vi "CRYGraph Polar Window.vi"() -> ()   [LabVIEW 2013]
uses:
  Control/CRYPolar Property.ctl
  Control/CRYFlag Cluster.ctl
  <vilib>/Utility/miscctls.llb/LVCursorListTypeDef.ctl
  <vilib>/Utility/miscctls.llb/LVRectTypeDef.ctl
  <vilib>/Utility/miscctls.llb/LVRowAndColumnTypeDef.ctl
  SubVI/CRYData View Global.vi
  CRYCurveLibrary/Global/CRYCurve Library Global.vi
  SubVI/CRYMain Sub Window Global.vi
panel:
  out "PhaseShow":bool=TRUE
  out "FrequencyVScrollShow":bool=TRUE
  out "LegendVScrollShow":bool=TRUE
  out "SelectedRow":i32[](array[numeric])
  out "Legend Ref":refnum<vi>
  in  "LoadFinish":bool
  in  "Legend 2":i32(listbox) caption="Legend"
  in  "AxisChange":bool
  out "MagnitudeShow":bool=TRUE
  in  "RemoveSome":bool
  in  "PaletteShow":bool
  in  "ScaleFitY 2":bool
  in  "ScaleFitY":bool
  in  "ScaleFitX":bool
  out "XY Graph Ref":refnum<vi>
  out "TotalPlotPolar":u32
  out "OldRowPolar":i32
  out "Repaint Watermark":i32
  out "PropertyTab":string
  out "Polar Plot":picture
  in  "stop":bool
  out "XYCursor":string
  in  "ColorBoxPolar":u32(colorbox)
  out "Event Name":string
  in  "Cursor":string[][](table)
  out "Queue Name":string
  out "Graph Ref":refnum<vi>
  out "Title Name":string
  out "OldRow":i32
  out "TotalPlot":u32
  out "Graph Number":i32
  in  "Frequency":i32(listbox) caption="Legend"
  out "XY Graph":cluster{"XY Graph":cluster{dbl, dbl}[]}[](graph)
  in  "OpenProperty":bool
  in  "RemoveAll":bool
  out "Test":string
  in  "ColorBox":u32(colorbox)
  in  "PropertyLoading":bool
  in  "Legend":i32[](listbox)
  in  "CursorShow":bool
  in  "LegendShow":bool
  out "Cursor Ref":refnum<vi>
  in  "StateOut":bool
  in  "XYShow":bool
  out "Polar Property":T1={"polar attributes"={"maximum"=2.0, "minimum"=0.0, "clip to min"=FALSE, "log"=FALSE, "grid color"=3381657, "plot color"=16711680, "fmt and prec"={"format"=enum."Decimal", "precision"=2}, "visible section"=4}, "Auto/Manual"=0, "Zero Adjust (deg)"=0, "Angle Increment (deg)"=0, "Mirror"=FALSE, "Auto Increment"=FALSE, "Total Rotatin (deg)"=0, "Discrete/Rannge"=0, "Show Name"=FALSE, "CurValues"=[], "CurIndex"=0, "CurColors"=[], "CurColors_Range"=[], "CurValues_Range"=[], "Pen"={"Width"=1, "Style"=enum."Solid"}, "BackgroundColor"=0} {"polar attributes"."minimum" format="%0.2f"; "polar attributes"."maximum" format="%0.2f"}
  in  "FrequencyShow":bool
  out "Frequency Ref":refnum<vi>
  in  "GraphType":string
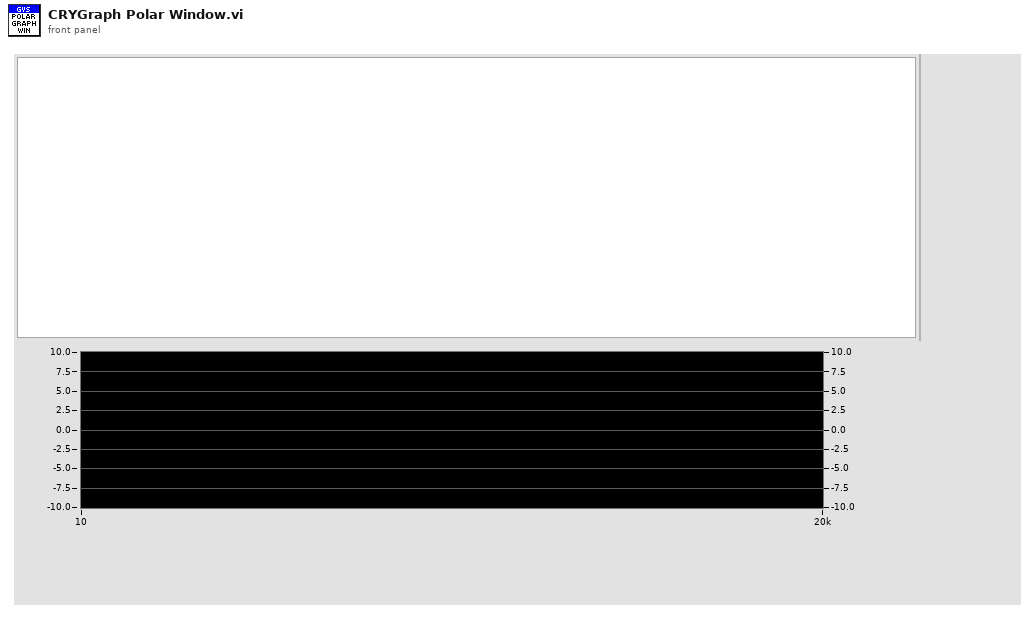
[diagram p1: front panel]
types:
  T1 = typedef "CRYPolar Property.ctl" = cluster{"polar attributes":cluster{"maximum":dbl, "minimum":dbl, "clip to min":bool, "log":bool, "grid color":u32, "plot color":u32, "fmt and prec":cluster{"format":enum8{"Decimal", "Scientific", "Engineering", "Binary", "Octal", "Hex"}, "precision":u8}, "visible section":u16}, "Auto/Manual":u16, "Zero Adjust (deg)":i32, "Angle Increment (deg)":i32, "Mirror":bool, "Auto Increment":bool, "Total Rotatin (deg)":i32, "Discrete/Rannge":u16, "Show Name":bool, "CurValues":dbl[], "CurIndex":u16, "CurColors":u32[], "CurColors_Range":u32[], "CurValues_Range":dbl[], "Pen":cluster{"Width":u16, "Style":enum32{"Solid", "Dash", "Dot", "DashDot", "DashDotDot"}}, "BackgroundColor":u32}
  T2 = typedef "CRYFlag Cluster.ctl" = cluster{"LegendShow":bool, "CellClick":bool, "Total Number":bool, "ScaleFitX":bool, "ScaleFitY":bool, "MapModeX":u8, "MapModeY":u8, "CursorShow":bool, "MagnitudeShow":bool, "PreviewShow":bool, "CursorEnabled":bool, "IntensityShow":bool, "PaletteShow":bool, "PhaseShow":bool, "XYShow":bool, "FrequencyShow":bool, "LegendVScrollShow":bool, "FrequencyVScrollShow":bool}
  T3 = enum32{"Solid", "Dash", "Dot", "DashDot", "DashDotDot"}
  T4 = enum8{"Decimal", "Scientific", "Engineering", "Binary", "Octal", "Hex"}
  T5 = typedef "LVCursorListTypeDef.ctl" = cluster{"Name":string, "Color":u32, "Style":u8, "Point Style":u8, "Name Visible":bool, "Allow Drag":bool, "Cursor Mode":u32, "Plot":i32, "Index":i32, "Position":cluster{"X":dbl, "Y":dbl}, "X Scale":u32, "Y Scale":u32, "Watch Plots":i32[], "Watch All Plots":bool, "Plot Area":i32, "Label Offset":cluster{"X":dbl, "Y":dbl}}[]
  T6 = typedef "CRYGraph Event.ctl" = cluster{"EvenName":string, "TitleName":string, "GraphName":string, "GraphType":string, "Data":variant, "Queue Name":string, "DataView Number":i32}
  T7 = typedef "LVBoundsTypeDef.ctl" = cluster{"Width":u32, "Height":u32}
  T8 = cluster{"maximum":dbl, "minimum":dbl, "clip to min":bool, "log":bool, "grid color":u32, "plot color":u32, "fmt and prec":cluster{"format":enum8{"Decimal", "Scientific", "Engineering", "Binary", "Octal", "Hex"}, "precision":u8}, "visible section":u16}
  T9 = enum16{"No Scaling", "Scale All Objects", "Scale Single Object"}
  T10 = cluster{"left":i16, "top":i16, "right":i16, "bottom":i16}
  T11 = typedef "LVRowAndColumnTypeDef.ctl" = cluster{"Row":i32, "Column":i32}
  T12 = cluster{"Name":string, "Color":u32, "Style":u8, "Point Style":u8, "Name Visible":bool, "Allow Drag":bool, "Cursor Mode":u32, "Plot":i32, "Index":i32, "Position":cluster{"X":dbl, "Y":dbl}, "X Scale":u32, "Y Scale":u32, "Watch Plots":i32[], "Watch All Plots":bool, "Plot Area":i32, "Label Offset":cluster{"X":dbl, "Y":dbl}}
  T13 = typedef "LVRectTypeDef.ctl" = cluster{"Left":i16, "Top":i16, "Right":i16, "Bottom":i16}
  T14 = typedef "LVPoint32TypeDef.ctl" = cluster{"Horizontal":i32, "Vertical":i32}
  T15 = typedef "LVPositionTypeDef.ctl" = cluster{"Left":i32, "Top":i32}
  T16 = typedef "CRYData Cluster.ctl" = cluster{"Name":string, "Curve":cluster{"x":dbl, "y":dbl, "z":dbl}[], "X data":u16, "Y data":u16, "Z data":u16, "X axis":u16, "Y axis":u16, "Z axis":u16, "X unit":string, "Y unit":string, "Z unit":string, "X dB ref":dbl, "Y dB ref":dbl, "Z dB ref":dbl, "single val":bool, "protected":bool, "display X":bool, "display Y":bool, "display Z":bool, "Test Info":string, "Step No.":i32, "Plot Settings":cluster{"Color":u32, "Interpolation":u8, "Point Style":u8, "Line Style":u8, "Point Color":u32, "Line Width":u8, "Bar Plot Style":u8, "Fill To":i16}, "AutoProtect":bool}
  T17 = cluster{"Name":string, "Color":u32, "Style":u8, "Point Style":u8, "Name Visible":bool, "Allow Drag":bool, "Cursor Mode":u32, "Plot":i32, "Index":i32, "Position":cluster{"X":dbl, "Y":dbl}, "X Scale":u32, "Y Scale":u32, "Watch Plots":i32[], "Watch All Plots":bool, "Plot Area":i32, "Label Offset":cluster{"X":dbl, "Y":dbl}}[]
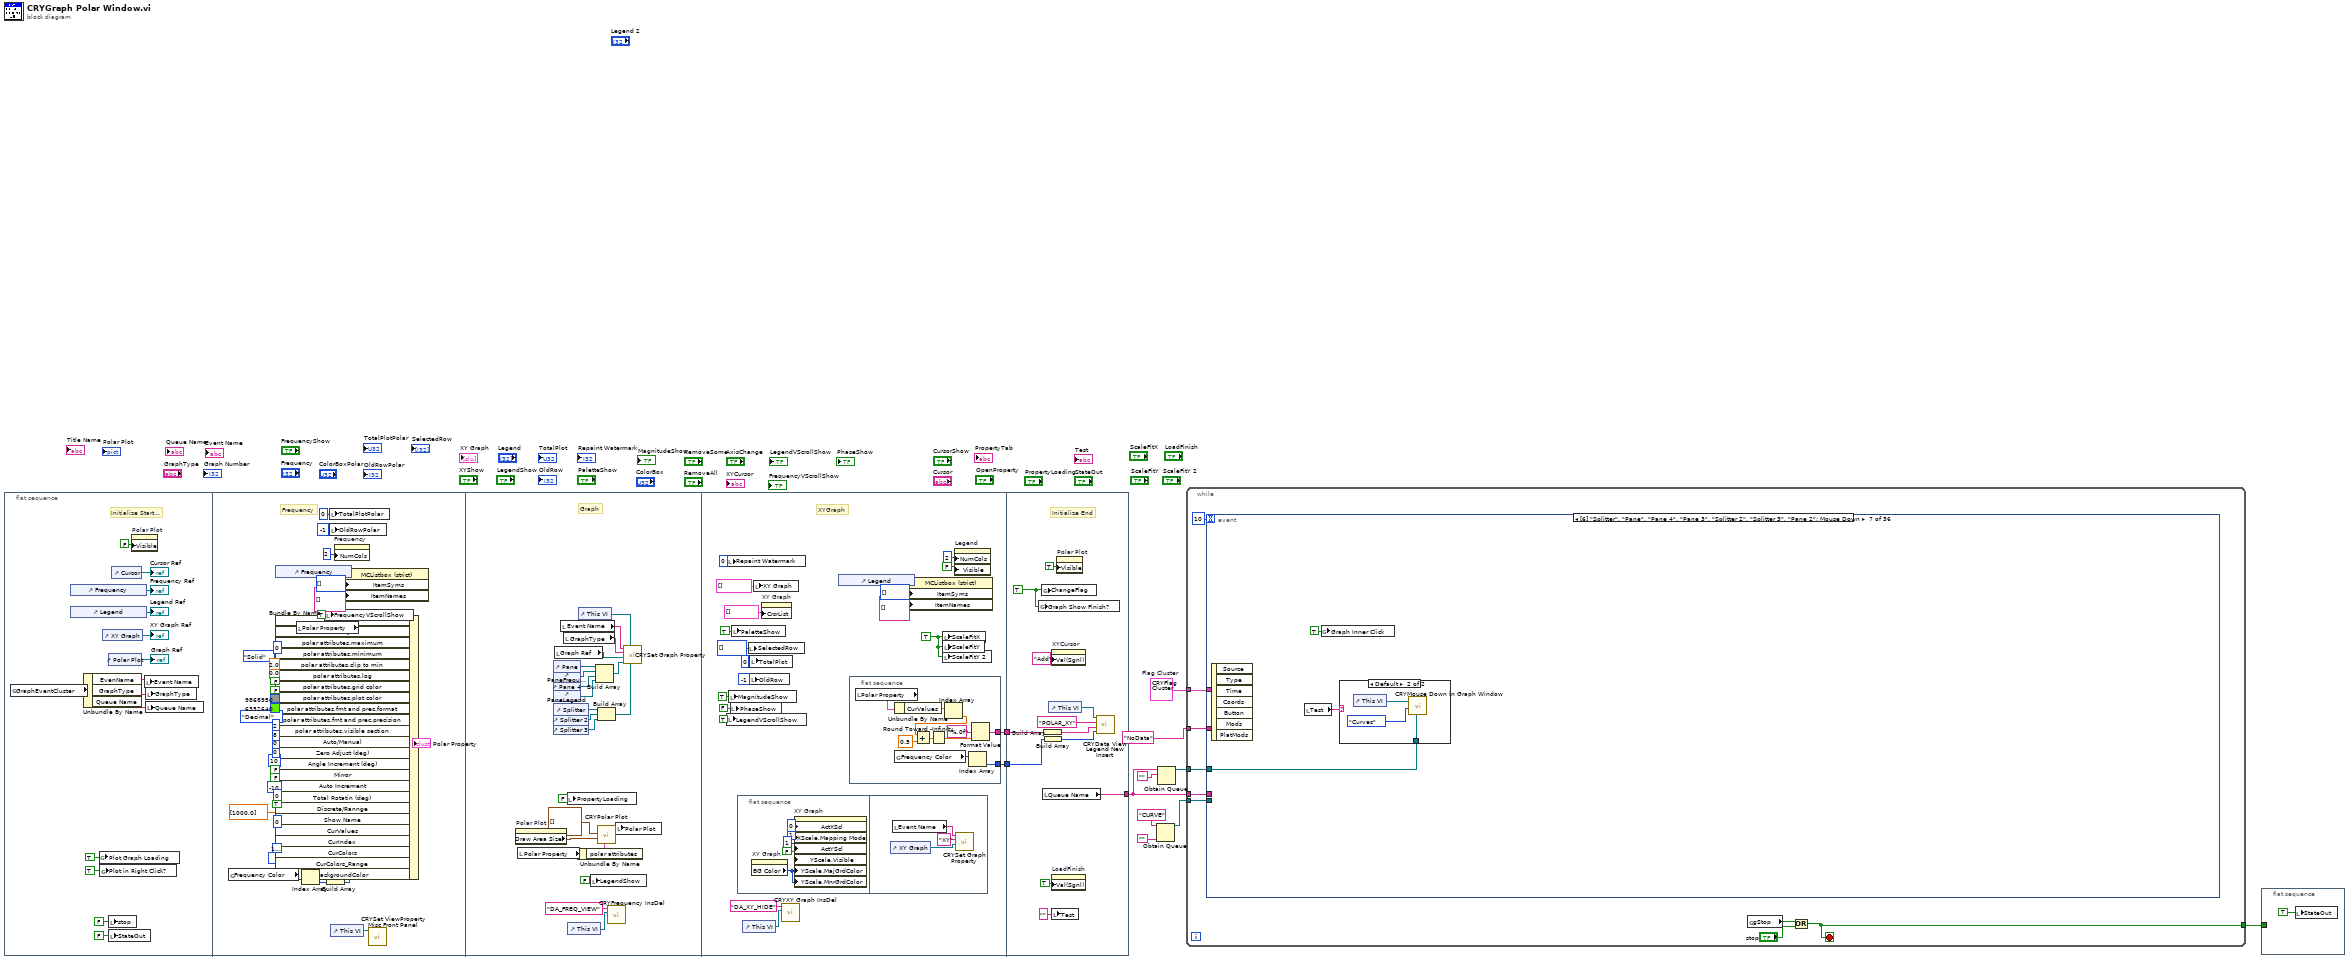
[diagram p0: block diagram]
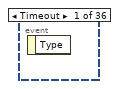
[diagram p2: hidden frame]
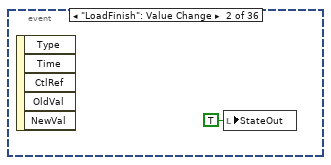
[diagram p3: hidden frame]
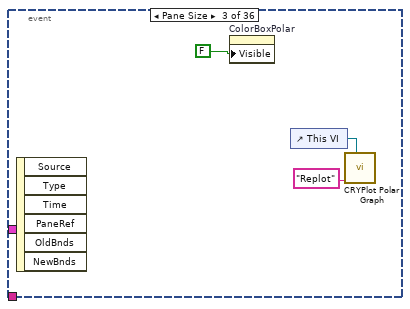
[diagram p4: hidden frame]
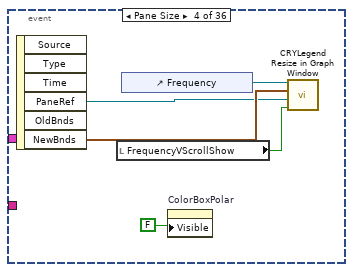
[diagram p5: hidden frame]
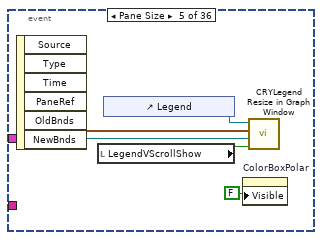
[diagram p6: hidden frame]
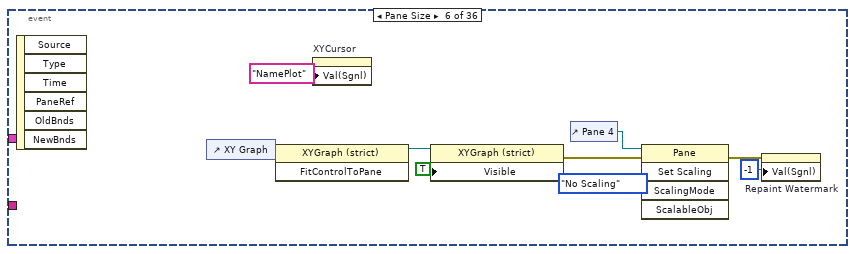
[diagram p7: hidden frame]
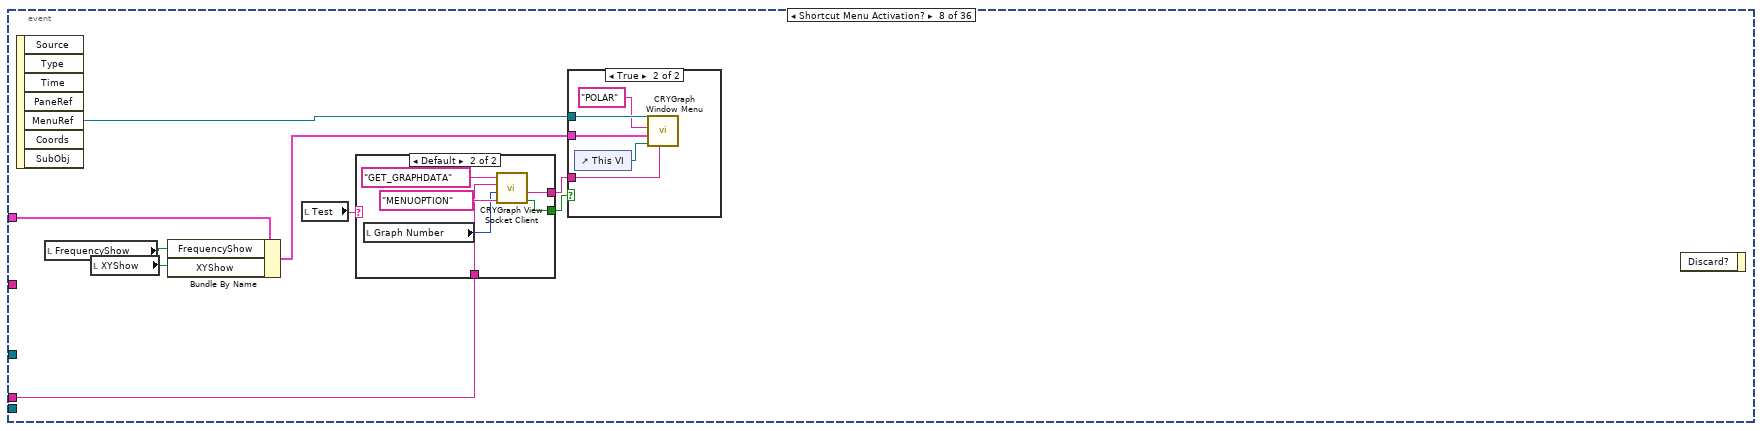
[diagram p9: hidden frame]
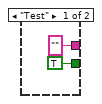
[diagram p10: hidden frame]
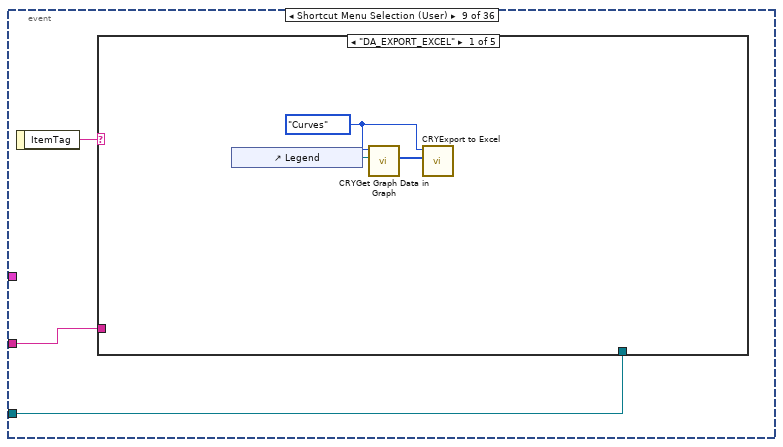
[diagram p12: hidden frame]
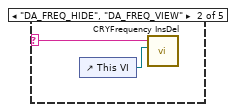
[diagram p13: hidden frame]
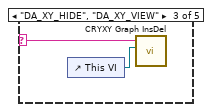
[diagram p14: hidden frame]
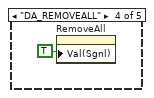
[diagram p15: hidden frame]
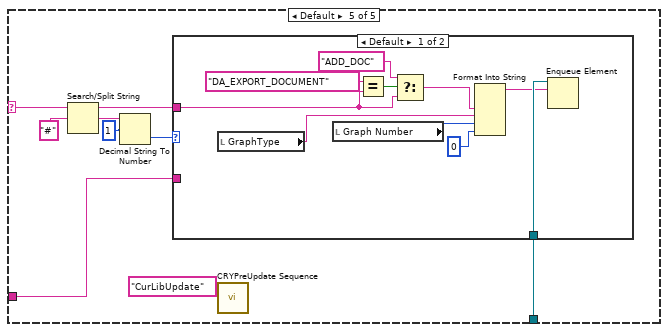
[diagram p16: hidden frame]
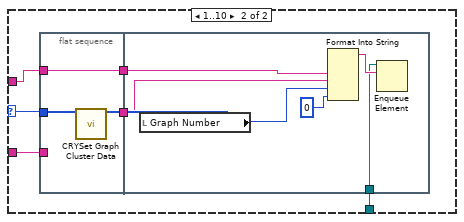
[diagram p17: hidden frame]
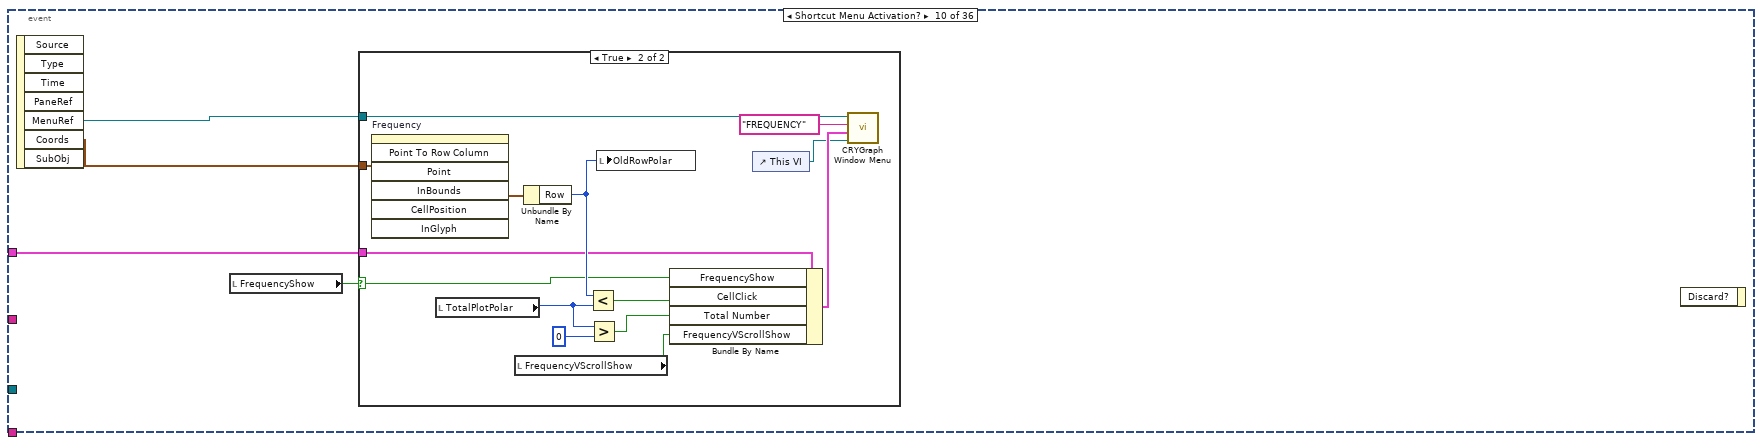
[diagram p18: hidden frame]
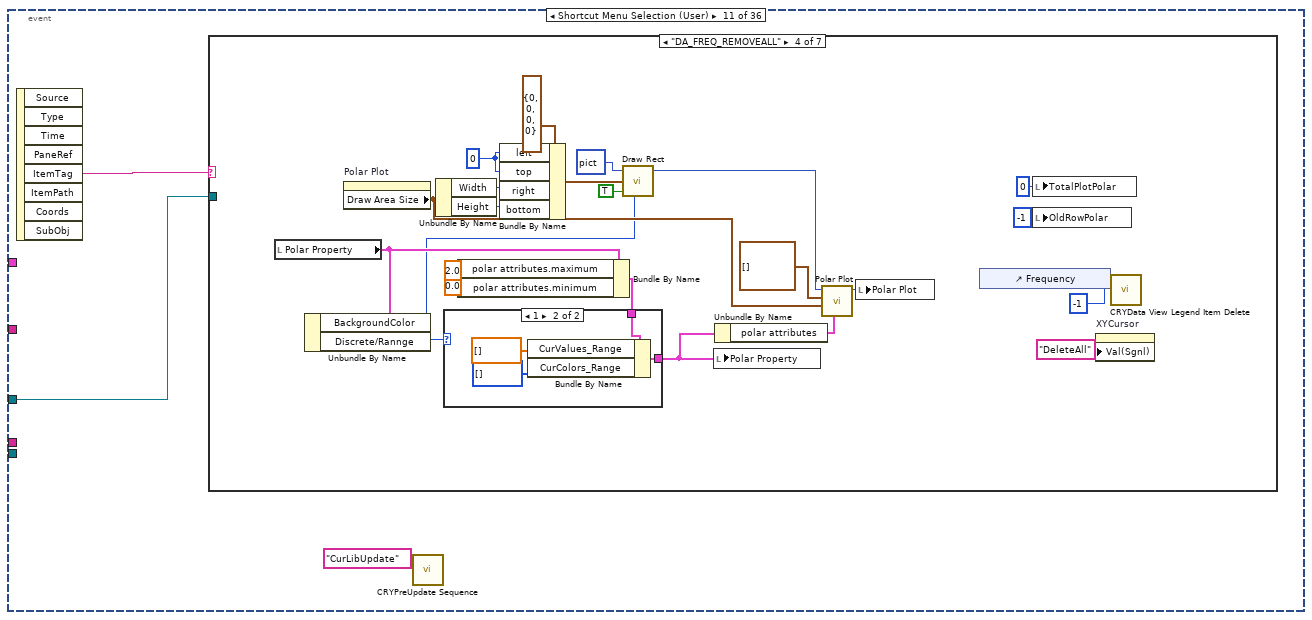
[diagram p20: hidden frame]
diagram:
  w9 = T2 {"LegendShow"=FALSE, "CellClick"=FALSE, "Total Number"=FALSE, "ScaleFitX"=FALSE, "ScaleFitY"=FALSE, "MapModeX"=0, "MapModeY"=0, "CursorShow"=FALSE, "MagnitudeShow"=FALSE, "PreviewShow"=FALSE, "CursorEnabled"=FALSE, "IntensityShow"=FALSE, "PaletteShow"=FALSE, "PhaseShow"=FALSE, "XYShow"=FALSE, "FrequencyShow"=FALSE, "LegendVScrollShow"=FALSE, "FrequencyVScrollShow"=FALSE}  # Flag Cluster
  n1 = flat-sequence {
    tunnel: [w87] -> w5
    tunnel: [w86] -> w4
    tunnel: [w129] -> w6
    tunnel: w5 -> [w127]
    tunnel: w4 -> [w125]
    frame #0 {
      # "Initialize Start..."
      n2 = global read "CRYData View Global.vi" "GraphEventCluster"() -> (w17:T6)
      n3 = control-ref of="Frequency"() -> (→"Frequency Ref":refnum<vi>)
      n4 = control-ref of="Legend"() -> (→"Legend Ref":refnum<vi>)
      n5 = Unbundle By Name(w17) -> ("EvenName"=w13:string, "GraphType"=w16:string, "Queue Name"=w18:string)
      n6 = global write "CRYData View Global.vi" "Plot Graph Loading"(TRUE ("Sequence Change for Replot")) -> ()
      n7 = global write "CRYData View Global.vi" "Plot in Right Click?"(TRUE ("Plot in Right Click?")) -> ()
      n8 = control-ref of="XY Graph"() -> (→"XY Graph Ref":refnum<vi>)
      n9 = control-ref of="Polar Plot"() -> (→"Graph Ref":refnum<vi>)
      n10 = local write "stop"(FALSE ("stop")) -> ()
      n11 = local write "StateOut"(FALSE ("StateOut")) -> ()
      n12 = control-ref of="Cursor"() -> (→"Cursor Ref":refnum<vi>)
      n13 = property on="Polar Plot" class="Pict"("Visible"=FALSE) -> ()  [unwired: 2 in, 2 out]
      n14 = local write "Event Name"(w13) -> ()
      n15 = local write "GraphType"(w16) -> ()
      n16 = local write "Queue Name"(w18) -> ()
    }
    frame #1 {
      # "Frequency"
      n17 = global read "CRYCurve Library Global.vi" "Frequency Color"() -> (w49:u32[])
      n18 = control-ref of="Frequency"() -> (w57:refnum<vi>)
      n19 = local read "Polar Property"() -> (w29:T1)
      n20 = Index Array(array=w49) -> (element=w50:u32)  [unwired: 1 in]
      n21 = local write "FrequencyVScrollShow"(TRUE ("FrequencyVScrollShow")) -> ()
      n22 = Build Array(w50) -> (w51:u32[])
      n23 = Bundle By Name(cluster=w29, "Pen.Width"=u16 0, "Pen.Style"=T3."Solid", "polar attributes.maximum"=2.0, "polar attributes.minimum"=0.0, "polar attributes.clip to min"=FALSE, "polar attributes.log"=FALSE, "polar attributes.grid color"=u32 9868950 ("grid color"), "polar attributes.plot color"=u32 6352640 ("plot color"), "polar attributes.fmt and prec.format"=T4."Decimal", "polar attributes.fmt and prec.precision"=u8 2, "polar attributes.visible section"=u16 8, "Auto/Manual"=u16 0, "Zero Adjust (deg)"=0, "Angle Increment (deg)"=10, "Mirror"=FALSE, "Auto Increment"=FALSE, "Total Rotatin (deg)"=-10, "Discrete/Rannge"=u16 0, "Show Name"=TRUE, "CurValues"=dbl[] [1000.0], "CurIndex"=u16 0, "CurColors"=w51, "CurColors_Range"=w51, "BackgroundColor"=u32 16777222 ("grid color")) -> (→"Polar Property":T1)
      n24 = local write "TotalPlotPolar"(u32 0 ("TotalPlotXY")) -> ()
      n25 = local write "OldRowPolar"(-1 ("OldRowXY")) -> ()
      n26 = control-ref of="This VI"() -> (w56:refnum<vi>)
      n27 = property on="Frequency" class="MCListbox (strict)"("NumCols"=u32 2 ("Number of Columns")) -> ()  [unwired: 2 in, 2 out]
      n28 = property on="Property Node" class="MCListbox (strict)"(reference=w57, "ItemSyms"=i32[] [] ("Item Symbols"), "ItemNames"=string[][] [] ("Item Names")) -> ()  [unwired: 1 in, 2 out]
      n29 = call "CRYSet ViewProperty Misc Front Panel.vi"("Vi Ref"=w56) -> ()  [unwired: 11 in]
    }
    frame #2 {
      # "Graph"
      n30 = property on="Polar Plot" class="Pict"() -> ("Draw Area Size"=w78:T7)  [unwired: 2 in, 2 out]
      n31 = local read "Polar Property"() -> (w82:T1)
      n32 = control-ref of="Pane"() -> (w67:refnum<vi>)
      n33 = control-ref of="PaneFrequency"() -> (w68:refnum<vi>)
      n34 = control-ref of="Pane 4"() -> (w71:refnum<vi>)
      n35 = control-ref of="PaneLegend"() -> (w72:refnum<vi>)
      n36 = control-ref of="Splitter"() -> (w69:refnum<vi>)
      n37 = control-ref of="Splitter 2"() -> (w70:refnum<vi>)
      n38 = control-ref of="Splitter 3"() -> (w73:refnum<vi>)
      n39 = local read "Graph Ref"() -> (w62:refnum<vi>)
      n40 = local read "Event Name"() -> (w66:string)
      n41 = local read "GraphType"() -> (w65:string)
      n42 = local write "PropertyLoading"(FALSE ("PropertyLoading")) -> ()
      n43 = control-ref of="This VI"() -> (w76:refnum<vi>)
      n44 = Unbundle By Name(w82) -> ("polar attributes"=w81:T8)
      n45 = control-ref of="This VI"() -> (w61:refnum<vi>)
      n46 = local write "LegendShow"(FALSE ("LegendShow")) -> ()
      n47 = Build Array(w67, w68, w71, w72) -> (w64:refnum<vi>[])
      n48 = call "CRYPolar Plot.vi"("polar attributes"=w81, "dimensions (w,h)"=w78, "data array [mag, phase (deg)]"=cluster{"magnitude":dbl, "phase":dbl}[] []) -> ("new picture"=w80:picture)  [unwired: 8 in]
      n49 = Build Array(w69, w70, w73) -> (w63:refnum<vi>[])
      n50 = call "CRYFrequency InsDel.vi"("Graph VI Ref"=w76, "sAction"="DA_FREQ_VIEW" ("Action Type")) -> ()  [unwired: 10 in]
      n51 = local write "Polar Plot"(w80) -> ()
      n52 = call "CRYSet Graph Property.vi"("Splitters"=w63, "pGraph VI In"=w61, "Panes"=w64, "Graph Ref"=w62, "Graph Type"=w65, "Event Name"=w66) -> ()  [unwired: 6 in]
    }
    frame #3 {
      w94 = TRUE ("ScaleFitX")
      # "XYGraph"
      n53 = local write "Repaint Watermark"(0 ("Repaint Watermark")) -> ()
      n54 = local write "LegendVScrollShow"(TRUE ("LegendVScrollShow")) -> ()
      n55 = local write "MagnitudeShow"(TRUE ("Magnitude")) -> ()
      n56 = local write "PhaseShow"(FALSE ("PhaseShow")) -> ()
      n57 = local write "PaletteShow"(TRUE ("PaletteShow")) -> ()
      n58 = flat-sequence {
        frame #0 {
          n59 = property on="XY Graph" class="XYGraph (strict)"() -> ("BG Color"=w105:u32)  [unwired: 2 in, 2 out]
          n60 = property on="XY Graph" class="XYGraph (strict)"("ActXScl"=0 ("Active X Scale"), "XScale.Mapping Mode"=u8 1 ("X Scale.Mapping Mode"), "ActYScl"=1 ("Active Y Scale"), "YScale.Visible"=FALSE ("Y Scale.Visible"), "YScale.MajGrdColor"=w105, "YScale.MnrGrdColor"=w105) -> ()  [unwired: 2 in, 2 out]
        }
        frame #1 {
          n61 = control-ref of="XY Graph"() -> (w108:refnum<vi>)
          n62 = local read "Event Name"() -> (w109:string)
          n63 = call "CRYSet Graph Property.vi"("Graph Ref"=w108, "Graph Type"="XY", "Event Name"=w109) -> ()  [unwired: 9 in]
        }
      }
      n64 = control-ref of="This VI"() -> (w100:refnum<vi>)
      n65 = local write "SelectedRow"(i32[] [] ("SelectedRow")) -> ()
      n66 = local write "OldRow"(-1 ("OldRow 2")) -> ()
      n67 = local write "TotalPlot"(u32 0 ("TotalPlot")) -> ()
      n68 = local write "XY Graph"(cluster{"XY Graph":cluster{dbl, dbl}[]}[] [] ("XY Graph")) -> ()
      n69 = property on="XY Graph" class="XYGraph (strict)"("CrsrList"=T5 [] ("Cursor List")) -> ()  [unwired: 2 in, 2 out]
      n70 = call "CRYXY Graph InsDel.vi"("Graph VI Ref"=w100, "sAction"="DA_XY_HIDE" ("Action Type")) -> ()  [unwired: 10 in]
      n71 = control-ref of="Legend"() -> (w89:refnum<vi>)
      n72 = flat-sequence {
        tunnel: [w113] -> w87
        tunnel: [w111] -> w86
        frame #0 {
          n73 = local read "Polar Property"() -> (w116:T1)
          n74 = Unbundle By Name(w116) -> ("CurValues"=w115:dbl[])
          n75 = global read "CRYCurve Library Global.vi" "Frequency Color"() -> (w112:u32[])
          n76 = Index Array(array=w115) -> (element=w114:dbl)  [unwired: 1 in]
          n77 = Add(x=w114, y=0.5) -> (x+y=w118:dbl)
          n78 = Round Toward -Infinity(1:w118) -> (0:w117:dbl)
          n79 = Index Array(array=w112) -> (element=w111:u32)  [unwired: 1 in]
          n80 = Format Value(format string="%.0f", value (0)=w117) -> (output string=w113:string)  [unwired: 1 in]
        }
      }
      n81 = property on="Property Node" class="MCListbox (strict)"(reference=w89, "ItemSyms"=i32[] [] ("Item Symbols"), "ItemNames"=string[][] [] ("Item Names")) -> ()  [unwired: 1 in, 2 out]
      n82 = local write "ScaleFitX"(w94) -> ()
      n83 = local write "ScaleFitY"(w94) -> ()
      n84 = local write "ScaleFitY 2"(w94) -> ()
      n85 = property on="Legend" class="MCListbox (strict)"("NumCols"=u32 2 ("Number of Columns"), "Visible"=FALSE) -> ()  [unwired: 2 in, 2 out]
    }
    frame #4 {
      w132 = TRUE ("ChangeFlag")
      # "Initialize End"
      n86 = global write "CRYData View Global.vi" "Graph Show Finish?"(w132) -> ()
      n87 = global write "CRYData View Global.vi" "ChangeFlag"(w132) -> ()
      n88 = local read "Queue Name"() -> (w129:string)
      n89 = Build Array(w127) -> (w126:string[])
      n90 = Build Array(w125) -> (w124:u32[])
      n91 = control-ref of="This VI"() -> (w121:refnum<vi>)
      n92 = property on="XYCursor" class="Str"("Val(Sgnl)"="Add" ("Value (Signaling)")) -> ()  [unwired: 2 in, 2 out]
      n93 = property on="LoadFinish" class="Bool (strict)"("Val(Sgnl)"=TRUE ("Value (Signaling)")) -> ()  [unwired: 2 in, 2 out]
      n94 = local write "Test"("" ("Test")) -> ()
      n95 = property on="Polar Plot" class="Pict"("Visible"=TRUE) -> ()  [unwired: 2 in, 2 out]
      n96 = call "CRYData View Legend New Insert.vi"("Color Array"=w124, "ItemName Array"=w126, "sOption"="POLAR_XY", "pGraph VI In"=w121) -> ()  [unwired: 2 in, 6 out]
    }
  }
  n97 = Obtain Queue(name (unnamed)="CURVE" ("YAxisTitle"), element data type="" ("Action Type")) -> (queue out=w1:refnum<queue>)  [unwired: 3 in, 2 out]
  n98 = Obtain Queue(name (unnamed)=w6, element data type="") -> (queue out=w11:refnum<queue>)  [unwired: 3 in, 2 out]
  n99 = while {
    tunnel: w11 -> [w141]
    tunnel: w9 -> [w137]
    tunnel: "NoData" ("input 2") -> [w135]
    tunnel: w6 -> [w136]
    tunnel: [w134] -> w7
    tunnel: w1 -> [w133]
    stop <- w134 stop-if-true
    n100 = event shown="[6] \"Splitter\", \"Pane\", \"Pane 4\", \"Pane 3\", \"Splitter 2\", \"Splitter 3\", \"Pane 2\": Mouse Down" {
      selector: _ -> [_ _ _ _ _ _ _ _ _ _ _ _ _ _ _ _ _ _ _ _ _ _ _ _ _ _ _ _ _ _ _ _ _ _ _ _]
      dyn-events: _ -> [_ _ _ _ _ _ _ _ _ _ _ _ _ _ _ _ _ _ _ _ _ _ _ _ _ _ _ _ _ _ _ _ _ _ _ _]
      timeout: 10 -> [_ _ _ _ _ _ _ _ _ _ _ _ _ _ _ _ _ _ _ _ _ _ _ _ _ _ _ _ _ _ _ _ _ _ _ _]
      tunnel: w141 -> [_ _ _ _ _ _ w167 _ w195 _ w257 _ w387 _ w488 _ _ _ _ _ _ _ _ _ _ _ _ _ _ _ _ _ _ _ _ w1235]
      tunnel: w137 -> [_ _ _ _ _ _ _ w178 _ w240 _ w364 _ w467 _ _ _ _ _ _ _ _ _ _ _ _ _ _ _ _ _ _ _ _ _ _]
      tunnel: w135 -> [_ _ _ _ _ _ _ _ w193 _ _ _ _ _ w487 _ _ _ _ _ _ _ _ _ _ _ _ _ _ _ _ _ _ _ _ _]
      tunnel: w136 -> [_ _ _ _ _ _ _ w173 _ _ _ w365 w386 _ _ _ _ _ _ _ _ _ _ _ _ _ _ _ _ _ _ _ _ _ _ _]
      tunnel: w133 -> [_ _ _ _ _ _ _ _ _ _ _ _ w385 _ _ _ _ _ _ _ _ _ _ _ _ _ _ _ _ _ _ _ _ _ _ _]
      event Timeout {
        n101 = event-data() -> ()  [unwired: 2 out]
      }
      event "LoadFinish": Value Change {
        n102 = event-data() -> ()  [unwired: 6 out]
        n103 = local write "StateOut"(TRUE ("StateOut")) -> ()
      }
      event Pane Size {
        n104 = event-data() -> ()  [unwired: 7 out]
        n105 = property on="ColorBoxPolar" class="ColBox"("Visible"=FALSE) -> ()  [unwired: 2 in, 2 out]
        n106 = control-ref of="This VI"() -> (w143:refnum<vi>)
        n107 = call "CRYPlot Polar Graph.vi"("pGraph VI In"=w143, "sOption"="Replot") -> ()  [unwired: 6 in, 4 out]
      }
      event Pane Size {
        n108 = event-data() -> ("PaneRef"=w149:refnum<vi>, "NewBnds"=w150:T13)  [unwired: 5 out]
        n109 = local read "FrequencyVScrollShow"() -> (w146:bool)
        n110 = control-ref of="Frequency"() -> (w147:refnum<vi>)
        n111 = property on="ColorBoxPolar" class="ColBox"("Visible"=FALSE) -> ()  [unwired: 2 in, 2 out]
        n112 = call "CRYLegend Resize in Graph Window.vi"("VScrollShow"=w146, "Pane Ref"=w149, "input cluster"=w150, "Legend"=w147) -> ()  [unwired: 8 out]
      }
      event Pane Size {
        n113 = event-data() -> ("PaneRef"=w154:refnum<vi>, "NewBnds"=w153:T13)  [unwired: 5 out]
        n114 = local read "LegendVScrollShow"() -> (w151:bool)
        n115 = control-ref of="Legend"() -> (w152:refnum<vi>)
        n116 = property on="ColorBoxPolar" class="ColBox"("Visible"=FALSE) -> ()  [unwired: 2 in, 2 out]
        n117 = call "CRYLegend Resize in Graph Window.vi"("VScrollShow"=w151, "Pane Ref"=w154, "input cluster"=w153, "Legend"=w152) -> ()  [unwired: 8 out]
      }
      event Pane Size {
        n118 = event-data() -> ()  [unwired: 7 out]
        n119 = control-ref of="XY Graph"() -> (w157:refnum<vi>)
        n120 = invoke class="XYGraph (strict)" method="FitControlToPane"(reference=w157) -> (reference out=w162:refnum<vi>)  [unwired: 2 in, 2 out]
        n121 = property on="XYCursor" class="Str"("Val(Sgnl)"="NamePlot" ("Value (Signaling)")) -> ()  [unwired: 2 in, 2 out]
        n122 = property class="XYGraph (strict)"(reference=w162, "Visible"=TRUE) -> (error out=w160:errorcluster)  [unwired: 1 in, 1 out]
        n123 = control-ref of="Pane 4"() -> (w158:refnum<vi>)
        n124 = invoke class="Pane" method="Set Scaling"(reference=w158, error in=w160, "ScalingMode"=T9."No Scaling" ("Scaling Mode")) -> (error out=w159:errorcluster)  [unwired: 2 in, 4 out]
        n125 = property on="Repaint Watermark" class="DigNum (strict)"(error in=w159, "Val(Sgnl)"=-1 ("Value (Signaling)")) -> ()  [unwired: 1 in, 2 out]
      }
      event Mouse Down {
        n126 = event-data() -> ()  [unwired: 8 out]
        n127 = local read "Test"() -> (w166:string)
        n128 = global write "CRYCurve Library Global.vi" "Graph Inner Click"(TRUE ("Graph Inner Click")) -> ()
        n129 = case shown="Default" w166 {
          tunnel: w167 -> [_ w169]
          frame "Test" {
          }
          frame Default {
            n130 = control-ref of="This VI"() -> (w168:refnum<vi>)
            n131 = call "CRYMouse Down in Graph Window.vi"("Queue"=w169, "Selected Type"=enum16{"Curves", "Values", "Results", "WFM"}."Curves" ("Type"), "pGraph VI In"=w168) -> ()  [unwired: 3 in, 6 out]
          }
        }
      }
      event Shortcut Menu Activation? {
        n132 = event-data() -> ("MenuRef"=w174:refnum<k9>)  [unwired: 7 out]
        n133 = local read "FrequencyShow"() -> (w179:bool)
        n134 = local read "XYShow"() -> (w171:bool)
        n135 = Bundle By Name(cluster=w178, "FrequencyShow"=w179, "XYShow"=w171) -> (w175:T2)
        n136 = local read "Test"() -> (w172:string)
        n137 = case shown="Default" w172 {
          tunnel: ["" ("sData Out") w185] -> w177
          tunnel: [TRUE ("bResult Out") w184] -> w176
          tunnel: w173 -> [_ w182]
          frame "Test" {
          }
          frame Default {
            n138 = local read "Graph Number"() -> (w183:i32)
            n139 = call "CRYGraph View Socket Client.vi"("sOption"="MENUOPTION", "nData"=w183, "sData"=w182, "sAction"="GET_GRAPHDATA") -> ("bResult Out"=w184:bool, "sData Out"=w185:string)  [unwired: 4 in, 2 out]
          }
        }
        n140 = case shown="True" w176 {
          tunnel: w174 -> [_ w192]
          tunnel: w175 -> [_ w190]
          tunnel: w177 -> [_ w189]
          frame False {
          }
          frame True {
            n141 = control-ref of="This VI"() -> (w188:refnum<vi>)
            n142 = call "CRYGraph Window Menu.vi"("MenuOption"=w189, "pGraph VI"=w188, "Flag Cluster"=w190, "Type"="POLAR", "Runtime Menu Ref In"=w192) -> ()  [unwired: 7 out]
          }
        }
        n143 = event-data() -> ()  [unwired: 2 in, 1 out]
      }
      event Shortcut Menu Selection (User) {
        n144 = event-data() -> ("ItemTag"=w194:string)  [unwired: 1 out]
        n145 = case shown="\"DA_EXPORT_EXCEL\"" w194 {
          selector: w194 -> [_ w199 w201 _ w206]
          tunnel: w195 -> [_ _ _ _ w207]
          tunnel: w193 -> [_ _ _ _ w205]
          frame "DA_EXPORT_EXCEL" {
            w196 = enum16{"Curves", "Values", "Results", "WFM"}."Curves" ("Type")
            n146 = control-ref of="Legend"() -> (w197:refnum<vi>)
            n147 = call "CRYGet Graph Data in Graph.vi"("Legend Refnum"=w197, "Type In"=w196) -> ("Rows"=w198:i32[])  [unwired: 2 in, 7 out]
            n148 = call "CRYExport to Excel.vi"("Rows"=w198, "Type"=w196) -> ()  [unwired: 2 in, 8 out]
          }
          frame "DA_FREQ_HIDE", "DA_FREQ_VIEW" {
            n149 = control-ref of="This VI"() -> (w200:refnum<vi>)
            n150 = call "CRYFrequency InsDel.vi"("Graph VI Ref"=w200, "sAction"=w199) -> ()  [unwired: 10 in]
          }
          frame "DA_XY_HIDE", "DA_XY_VIEW" {
            n151 = control-ref of="This VI"() -> (w202:refnum<vi>)
            n152 = call "CRYXY Graph InsDel.vi"("Graph VI Ref"=w202, "sAction"=w201) -> ()  [unwired: 10 in]
          }
          frame "DA_REMOVEALL" {
            n153 = property on="RemoveAll" class="Bool (strict)"("Val(Sgnl)"=TRUE ("Value (Signaling)")) -> ()  [unwired: 2 in, 2 out]
          }
          frame Default {
            n154 = Search/Split String(string=w206, search string/char (-)="#") -> (substring before match=w212:string, match + rest of string=w209:string)  [unwired: 2 out]
            n155 = Decimal String To Number(string=w209, offset=1) -> (number=w211:i32)  [unwired: 2 out]
            n156 = case shown="Default" w211 {
              selector: w211 -> [_ w225]
              tunnel: w212 -> [w215 w228]
              tunnel: w207 -> [w222 w227]
              tunnel: w205 -> [_ w223]
              frame Default {
                n157 = local read "GraphType"() -> (w213:string)
                n158 = local read "Graph Number"() -> (w219:i32)
                n159 = Equal?(x="DA_EXPORT_DOCUMENT" ("y"), y=w215) -> (x = y?=w218:bool)
                n160 = Select(t="ADD_DOC", s=w218, f=w215) -> (s? t:f=w214:string)
                n161 = Format Into String(w214, w213, w219, 0 ("input 3")) -> (resulting string=w221:string)  [unwired: 3 in, 1 out]
                n162 = Enqueue Element(queue=w222, element=w221) -> ()  [unwired: 1 in, 4 out]
              }
              frame 1..10 {
                n163 = flat-sequence {
                  tunnel: w228 -> [w231]
                  tunnel: [w231] -> w226
                  tunnel: w225 -> [w230]
                  tunnel: [w229] -> w224
                  tunnel: w223 -> [_]
                  tunnel: w227 -> [w235]
                  tunnel: w226 -> [w234]
                  tunnel: w224 -> [w233]
                  frame #0 {
                    n164 = call "CRYSet Graph Cluster Data.vi"("Graph Number"=w230) -> ("DataType"=w229:string)  [unwired: 2 in, 8 out]
                  }
                  frame #1 {
                    n165 = local read "Graph Number"() -> (w232:i32)
                    n166 = Format Into String(w234, w233, w232, 0 ("input 3")) -> (resulting string=w237:string)  [unwired: 3 in, 1 out]
                    n167 = Enqueue Element(queue=w235, element=w237) -> ()  [unwired: 1 in, 4 out]
                  }
                }
              }
            }
            n168 = call "CRYPreUpdate Sequence.vi"("EventName"="CurLibUpdate") -> ()  [unwired: 15 in]
          }
        }
      }
      event Shortcut Menu Activation? {
        n169 = event-data() -> ("MenuRef"=w241:refnum<k9>, "Coords"=w239:T14)  [unwired: 6 out]
        n170 = local read "FrequencyShow"() -> (w238:bool)
        n171 = case shown="True" w238 {
          selector: w238 -> [_ w243]
          tunnel: w241 -> [_ w251]
          tunnel: w240 -> [_ w249]
          tunnel: w239 -> [_ w247]
          frame False {
          }
          frame True {
            n172 = invoke on="Frequency" class="MCListbox (strict)" method="Point To Row Column"("Point"=w247) -> ("CellPosition"=w246:T11)  [unwired: 6 in, 6 out]
            n173 = local read "TotalPlotPolar"() -> (w248:u32)
            n174 = local read "FrequencyVScrollShow"() -> (w242:bool)
            n175 = Unbundle By Name(w246) -> ("Row"=w250:i32)
            n176 = Less?(x=w250, y=w248) -> (x < y?=w254:bool)
            n177 = Greater?(x=w248, y=u32 0) -> (0:w255:bool)
            n178 = local write "OldRowPolar"(w250) -> ()
            n179 = Bundle By Name(cluster=w249, "FrequencyShow"=w243, "CellClick"=w254, "Total Number"=w255, "FrequencyVScrollShow"=w242) -> (w245:T2)
            n180 = control-ref of="This VI"() -> (w244:refnum<vi>)
            n181 = call "CRYGraph Window Menu.vi"("pGraph VI"=w244, "Flag Cluster"=w245, "Type"="FREQUENCY", "Runtime Menu Ref In"=w251) -> ()  [unwired: 1 in, 7 out]
          }
        }
        n182 = event-data() -> ()  [unwired: 2 in, 1 out]
      }
      event Shortcut Menu Selection (User) {
        n183 = event-data() -> ("ItemTag"=w258:string)  [unwired: 8 out]
        n184 = case shown="\"DA_FREQ_REMOVEALL\"" w258 {
          selector: w258 -> [_ _ _ _ _ _ w356]
          tunnel: w257 -> [_ _ _ _ _ _ _]
          frame Default {
          }
          frame "DA_FREQ_HIDE_1" {
            n185 = control-ref of="This VI"() -> (w259:refnum<vi>)
            n186 = call "CRYFrequency InsDel.vi"("Graph VI Ref"=w259, "sAction"="DA_FREQ_HIDE") -> ()  [unwired: 10 in]
          }
          frame "DA_FREQ_REMOVE" {
            n187 = flat-sequence {
              tunnel: [w262] -> w261
              tunnel: w261 -> [w304]
              frame #0 {
                n188 = local read "TotalPlotPolar"() -> (w268:u32)
                n189 = local read "Polar Property"() -> (w263:T1)
                n190 = Decrement(x=w268) -> (x-1=w265:u32)
                n191 = control-ref of="Frequency"() -> (w267:refnum<vi>)
                n192 = local write "TotalPlotPolar"(w265) -> ()
                n193 = Unbundle By Name(w263) -> ("Discrete/Rannge"=w262:u16)
                n194 = local read "OldRowPolar"() -> (w264:i32)
                n195 = call "CRYData View Legend Item Delete.vi"("RowNumber"=w264, "Legend MultiListbox In"=w267) -> ()  [unwired: 10 out]
                n196 = case shown="0, Default" w262 {
                  tunnel: w263 -> [w272 w289]
                  tunnel: [w271 w288] -> w266
                  tunnel: w265 -> [w270 w287]
                  tunnel: w264 -> [w269 w286]
                  frame 0, Default {
                    n197 = case shown="1, Default" w270 {
                      tunnel: w272 -> [w275 w285]
                      tunnel: [w274 w284] -> w271
                      tunnel: w269 -> [_ w279]
                      frame 0 {
                        n198 = Bundle By Name(cluster=w275, "polar attributes.maximum"=1.0, "polar attributes.minimum"=-1.0, "CurValues"=dbl[] [], "CurColors"=u32[] []) -> (w274:T1)
                      }
                      frame 1, Default {
                        n199 = Unbundle By Name(w285) -> ("CurValues"=w283:dbl[], "CurColors"=w281:u32[])
                        n200 = Delete From Array(array=w283, index=w279) -> (array with subset deleted=w282:dbl[])  [unwired: 1 in, 1 out]
                        n201 = Delete From Array(array=w281, index=w279) -> (array with subset deleted=w280:u32[])  [unwired: 1 in, 1 out]
                        n202 = Bundle By Name(cluster=w285, "CurValues"=w282, "CurColors"=w280) -> (w284:T1)
                      }
                    }
                  }
                  frame 1 {
                    n203 = case shown="1, Default" w287 {
                      tunnel: w289 -> [w292 w302]
                      tunnel: [w291 w301] -> w288
                      tunnel: w286 -> [_ w296]
                      frame 0 {
                        n204 = Bundle By Name(cluster=w292, "polar attributes.maximum"=1.0, "polar attributes.minimum"=-1.0, "CurValues"=dbl[] [], "CurColors"=u32[] []) -> (w291:T1)
                      }
                      frame 1, Default {
                        n205 = Unbundle By Name(w302) -> ("CurValues_Range"=w300:dbl[], "CurColors_Range"=w298:u32[])
                        n206 = Delete From Array(array=w300, index=w296) -> (array with subset deleted=w299:dbl[])  [unwired: 1 in, 1 out]
                        n207 = Delete From Array(array=w298, index=w296) -> (array with subset deleted=w297:u32[])  [unwired: 1 in, 1 out]
                        n208 = Bundle By Name(cluster=w302, "CurValues_Range"=w299, "CurColors_Range"=w297) -> (w301:T1)
                      }
                    }
                  }
                }
                n209 = local write "Polar Property"(w266) -> ()
              }
              frame #1 {
                n210 = control-ref of="This VI"() -> (w303:refnum<vi>)
                n211 = case shown="0, Default" w304 {
                  frame 0, Default {
                    n212 = property on="XYCursor" class="Str"("Val(Sgnl)"="DeleteSelf" ("Value (Signaling)")) -> ()  [unwired: 2 in, 2 out]
                  }
                  frame 1 {
                  }
                }
                n213 = call "CRYPlot Polar Graph.vi"("pGraph VI In"=w303, "sOption"="Replot") -> ()  [unwired: 6 in, 4 out]
              }
            }
          }
          frame "DA_FREQ_REMOVEALL" {
            w314 = i16 0 ("left")
            n214 = local read "Polar Property"() -> (w323:T1)
            n215 = Unbundle By Name(w323) -> ("BackgroundColor"=w307:u32, "Discrete/Rannge"=w320:u16)
            n216 = property on="Polar Plot" class="Pict"() -> ("Draw Area Size"=w308:T7)  [unwired: 2 in, 2 out]
            n217 = Unbundle By Name(w308) -> ("Width"=w315:u32, "Height"=w316:u32)
            n218 = Bundle By Name(cluster=w323, "polar attributes.maximum"=2.0, "polar attributes.minimum"=0.0) -> (w319:T1)
            n219 = case shown="1" w320 {
              tunnel: [w332 w336] -> w318
              tunnel: w319 -> [w331 w335]
              frame 0, Default {
                n220 = Bundle By Name(cluster=w331, "CurValues"=dbl[] [], "CurColors"=u32[] []) -> (w332:T1)
              }
              frame 1 {
                n221 = Bundle By Name(cluster=w335, "CurValues_Range"=dbl[] [] ("CurValues"), "CurColors_Range"=u32[] [] ("CurColors")) -> (w336:T1)
              }
            }
            n222 = Bundle By Name(cluster=T10 {"left"=0, "top"=0, "right"=0, "bottom"=0} ("rect"), "left"=w314, "top"=w314, "right"=w315, "bottom"=w316) -> (w310:T10)
            n223 = call <vilib>:"Draw Rect.vi"("picture"=picture data[5B] ("Value"), "rect"=w310, "fill?(F)"=TRUE, "color(black)"=w307) -> ("new picture"=w309:picture)  [unwired: 5 in]
            n224 = local write "Polar Property"(w318) -> ()
            n225 = Unbundle By Name(w318) -> ("polar attributes"=w329:T8)
            n226 = call <vilib>:"Polar Plot.vi"("polar attributes"=w329, "dimensions (w,h)"=w308, "data array [mag, phase (deg)]"=cluster{"magnitude":dbl, "phase":dbl}[] [], "picture"=w309) -> ("new picture"=w328:picture)  [unwired: 7 out]
            n227 = local write "Polar Plot"(w328) -> ()
            n228 = control-ref of="Frequency"() -> (w324:refnum<vi>)
            n229 = local write "TotalPlotPolar"(u32 0 ("TotalPlot")) -> ()
            n230 = local write "OldRowPolar"(-1 ("OldRow 2")) -> ()
            n231 = property on="XYCursor" class="Str"("Val(Sgnl)"="DeleteAll" ("Value (Signaling)")) -> ()  [unwired: 2 in, 2 out]
            n232 = call "CRYData View Legend Item Delete.vi"("RowNumber"=-1, "Legend MultiListbox In"=w324) -> ()  [unwired: 10 out]
          }
          frame "DA_FREQ_INVERT" {
            n233 = flat-sequence {
              frame #0 {
                n234 = property on="Frequency" class="MCListbox (strict)"() -> ("ItemSyms"=w340:i32[])  [unwired: 2 in, 2 out]
                n235 = for {
                  tunnel: w340 -> [w345] mode=indexing
                  tunnel: [w341] -> w339 mode=indexing
                  w342 = 38
                  n236 = Equal?(x=w345, y=w342) -> (x = y?=w344:bool)
                  n237 = Select(t=37, s=w344, f=w342) -> (s? t:f=w341:i32)
                }
                n238 = property on="Frequency" class="MCListbox (strict)"("ItemSyms"=w339) -> ()  [unwired: 2 in, 2 out]
              }
              frame #1 {
                n239 = control-ref of="This VI"() -> (w346:refnum<vi>)
                n240 = property on="XYCursor" class="Str"("Val(Sgnl)"="Invert" ("Value (Signaling)")) -> ()  [unwired: 2 in, 2 out]
                n241 = call "CRYPlot Polar Graph.vi"("pGraph VI In"=w346, "sOption"="Replot") -> ()  [unwired: 6 in, 4 out]
              }
            }
          }
          frame "DA_FREQ_SHOWALL" {
            n242 = flat-sequence {
              frame #0 {
                n243 = property on="Frequency" class="MCListbox (strict)"() -> ("ItemSyms"=w350:i32[])  [unwired: 2 in, 2 out]
                n244 = for {
                  tunnel: w350 -> [_] mode=indexing
                  tunnel: [38] -> w349 mode=indexing
                }
                n245 = property on="Frequency" class="MCListbox (strict)"("ItemSyms"=w349) -> ()  [unwired: 2 in, 2 out]
              }
              frame #1 {
                n246 = control-ref of="This VI"() -> (w352:refnum<vi>)
                n247 = property on="XYCursor" class="Str"("Val(Sgnl)"="ShowAll" ("Value (Signaling)")) -> ()  [unwired: 2 in, 2 out]
                n248 = call "CRYPlot Polar Graph.vi"("pGraph VI In"=w352, "sOption"="Replot") -> ()  [unwired: 6 in, 4 out]
              }
            }
          }
          frame "DA_FREQ_VSCROLL_HIDE", "DA_FREQ_VSCROLL_VIEW" {
            n249 = Equal?(x="DA_FREQ_VSCROLL_VIEW" ("y"), y=w356) -> (x = y?=w355:bool)
            n250 = property on="FrequencyVScrollShow" class="Bool (strict)"("Val(Sgnl)"=w355) -> ()  [unwired: 2 in, 2 out]
          }
        }
        n251 = call "CRYPreUpdate Sequence.vi"("EventName"="CurLibUpdate") -> ()  [unwired: 15 in]
      }
      event Shortcut Menu Activation? {
        n252 = event-data() -> ("MenuRef"=w366:refnum<k9>)  [unwired: 7 out]
        n253 = property on="XY Graph" class="XYGraph (strict)"() -> ("XScale.Mapping Mode"=w359:u8, "YScale.Mapping Mode"=w358:u8)  [unwired: 2 in, 2 out]
        n254 = local read "LegendShow"() -> (w367:bool)
        n255 = local read "PaletteShow"() -> (w362:bool)
        n256 = local read "ScaleFitX"() -> (w361:bool)
        n257 = local read "ScaleFitY"() -> (w360:bool)
        n258 = local read "XYShow"() -> (w363:bool)
        n259 = Bundle By Name(cluster=w364, "XYShow"=w363, "LegendShow"=w367, "PaletteShow"=w362, "ScaleFitX"=w361, "ScaleFitY"=w360, "MapModeX"=w359, "MapModeY"=w358) -> (w369:T2)
        n260 = local read "Test"() -> (w368:string)
        n261 = case shown="Default" w368 {
          tunnel: ["" ("sData Out") w377] -> w371
          tunnel: [TRUE ("bResult Out") w376] -> w370
          tunnel: w365 -> [_ w374]
          frame "Test" {
          }
          frame Default {
            n262 = local read "Graph Number"() -> (w375:i32)
            n263 = call "CRYGraph View Socket Client.vi"("sOption"="MENUOPTION", "nData"=w375, "sData"=w374, "sAction"="GET_GRAPHDATA") -> ("bResult Out"=w376:bool, "sData Out"=w377:string)  [unwired: 4 in, 2 out]
          }
        }
        n264 = case shown="True" w370 {
          tunnel: w366 -> [_ w384]
          tunnel: w369 -> [_ w382]
          tunnel: w371 -> [_ w381]
          frame False {
          }
          frame True {
            n265 = control-ref of="This VI"() -> (w380:refnum<vi>)
            n266 = call "CRYGraph Window Menu.vi"("MenuOption"=w381, "pGraph VI"=w380, "Flag Cluster"=w382, "Type"="POLAR_XY", "Runtime Menu Ref In"=w384) -> ()  [unwired: 7 out]
          }
        }
        n267 = event-data() -> ()  [unwired: 2 in, 1 out]
      }
      event Shortcut Menu Selection (User) {
        n268 = event-data() -> ("ItemTag"=w388:string)  [unwired: 1 out]
        n269 = case shown="\"DA_EXPORT_EXCEL\"" w388 {
          selector: w388 -> [w390 _ w437 _ w450 w454 _ _]
          tunnel: w386 -> [_ _ _ _ _ _ _ w458]
          tunnel: w387 -> [_ _ w446 _ _ _ _ _]
          tunnel: w385 -> [_ _ _ _ _ _ _ w459]
          frame "DA_SCALE_X_A", "DA_SCALE_X_L", "DA_SCALE_Y_A", "DA_SCALE_Y_L" {
            n270 = case shown="\"DA_SCALE_Y_L\"" w390 {
              selector: w390 -> [w395 w408 w412 w433]
              tunnel: [w395 w408 w412 w433] -> w389
              frame "DA_SCALE_X_A", Default {
                n271 = local read "ScaleFitX"() -> (w394:bool)
                n272 = Not(x=w394) -> (.not. x?=w393:bool)
                n273 = Select(t=u8 2, s=w393, f=u8 0) -> (s? t:f=w396:u8)
                n274 = property on="XY Graph" class="XYGraph (strict)"("XScale.ScaleFit"=w396) -> ()  [unwired: 2 in, 2 out]
                n275 = local write "ScaleFitX"(w393) -> ()
              }
              frame "DA_SCALE_Y_A" {
                n276 = local read "ScaleFitY"() -> (w400:bool)
                n277 = local read "ScaleFitY 2"() -> (w402:bool)
                n278 = Not(x=w400) -> (.not. x?=w399:bool)
                n279 = Not(x=w402) -> (.not. x?=w401:bool)
                n280 = Select(t=u8 2, s=w401, f=u8 0) -> (s? t:f=w405:u8)
                n281 = Select(t=u8 2, s=w399, f=u8 0) -> (s? t:f=w409:u8)
                n282 = local write "ScaleFitY"(w399) -> ()
                n283 = property on="XY Graph" class="XYGraph (strict)"("ActYScl"=1 ("Active Y Scale"), "YScale.ScaleFit"=w405) -> ()  [unwired: 2 in, 2 out]
                n284 = property on="XY Graph" class="XYGraph (strict)"("ActYScl"=0 ("Active Y Scale"), "YScale.ScaleFit"=w409) -> ()  [unwired: 2 in, 2 out]
                n285 = local write "ScaleFitY 2"(w401) -> ()
              }
              frame "DA_SCALE_X_L" {
                n286 = property on="XY Graph" class="XYGraph (strict)"() -> ("XScale.Mapping Mode"=w413:u8)  [unwired: 2 in, 2 out]
                n287 = Equal?(x=w413, y=u8 0) -> (x = y?=w418:bool)
                n288 = Select(t=u8 1, s=w418, f=u8 0) -> (s? t:f=w414:u8)
                n289 = property on="XY Graph" class="XYGraph (strict)"("XScale.Mapping Mode"=w414) -> ()  [unwired: 2 in, 2 out]
              }
              frame "DA_SCALE_Y_L" {
                n290 = property on="XY Graph" class="XYGraph (strict)"("ActYScl"=0 ("Active Y Scale")) -> ("YScale.Mapping Mode"=w432:u8)  [unwired: 2 in, 2 out]
                n291 = property on="XY Graph" class="XYGraph (strict)"("ActYScl"=1 ("Active Y Scale")) -> ("YScale.Mapping Mode"=w419:u8)  [unwired: 2 in, 2 out]
                n292 = Equal To 0?(x=w432) -> (x = 0?=w426:bool)
                n293 = Equal To 0?(x=w419) -> (x = 0?=w425:bool)
                n294 = Select(t=u8 1, s=w426, f=u8 0) -> (s? t:f=w429:u8)
                n295 = Select(t=u8 1, s=w425, f=u8 0) -> (s? t:f=w422:u8)
                n296 = property on="XY Graph" class="XYGraph (strict)"("ActYScl"=0 ("Active Y Scale"), "YScale.Mapping Mode"=w429) -> ()  [unwired: 2 in, 2 out]
                n297 = property on="XY Graph" class="XYGraph (strict)"("ActYScl"=1 ("Active Y Scale"), "YScale.Mapping Mode"=w422) -> ()  [unwired: 2 in, 2 out]
              }
            }
            n298 = disable-structure shown="Disabled" {
              disable-tunnel: w389 -> [w391 _]
              frame Disabled {
                n299 = case shown="\"DA_SCALE_X_A\", \"DA_SCALE_Y_A\"" w391 {
                  frame Default {
                  }
                  frame "DA_SCALE_X_A", "DA_SCALE_Y_A" {
                    n300 = property on="Property Node" class="Bool (strict)"("Val(Sgnl)"=TRUE ("Value (Signaling)")) -> ()  [unwired: 2 in, 2 out]
                  }
                }
              }
              frame Enabled {
              }
            }
          }
          frame "DA_EXPORT_EXCEL" {
            w435 = enum16{"Curves", "Values", "Results", "WFM"}."Curves" ("Type")
            n301 = control-ref of="Legend"() -> (w434:refnum<vi>)
            n302 = call "CRYGet Graph Data in Graph.vi"("Legend Refnum"=w434, "Type In"=w435) -> ("Rows"=w436:i32[])  [unwired: 2 in, 7 out]
            n303 = call "CRYExport to Excel.vi"("Rows"=w436, "Type"=w435) -> ()  [unwired: 2 in, 8 out]
          }
          frame Default {
            n304 = call "CRYPreUpdate Sequence.vi"("EventName"="CurLibUpdate") -> ()  [unwired: 15 in]
            n305 = local read "Graph Number"() -> (w443:i32)
            n306 = local read "GraphType"() -> (w442:string)
            n307 = Equal?(x="DA_EXPORT_DOCUMENT" ("y"), y=w437) -> (x = y?=w441:bool)
            n308 = Select(t="ADD_DOC", s=w441, f=w437) -> (s? t:f=w438:string)
            n309 = Format Into String(w438, w442, w443, 0 ("input 3")) -> (resulting string=w444:string)  [unwired: 3 in, 1 out]
            n310 = Enqueue Element(queue=w446, element=w444) -> ()  [unwired: 1 in, 4 out]
          }
          frame "DA_XY_HIDE_1" {
            n311 = control-ref of="This VI"() -> (w448:refnum<vi>)
            n312 = call "CRYXY Graph InsDel.vi"("Graph VI Ref"=w448, "sAction"="DA_XY_HIDE") -> ()  [unwired: 10 in]
          }
          frame "DA_LEG_HIDE", "DA_LEG_VIEW" {
            n313 = control-ref of="This VI"() -> (w451:refnum<vi>)
            n314 = call "CRYData View Legend InsDel.vi"("sOption"="Polar_XY_Legend", "Graph VI Ref"=w451, "sAction"=w450) -> ()  [unwired: 1 in, 8 out]
          }
          frame "DA_PAL_HIDE", "DA_PAL_VIEW" {
            n315 = Equal?(x="DA_PAL_VIEW", y=w454) -> (x = y?=w453:bool)
            n316 = local write "PaletteShow"(w453) -> ()
            n317 = property on="XY Graph" class="XYGraph (strict)"("Palette Visible"=w453) -> ()  [unwired: 2 in, 2 out]
          }
          frame "DA_REMOVEALL" {
            n318 = property on="RemoveAll" class="Bool (strict)"("Val(Sgnl)"=TRUE ("Value (Signaling)")) -> ()  [unwired: 2 in, 2 out]
          }
          frame "DA_PROPERTY" {
            n319 = local read "Test"() -> (w457:string)
            n320 = case shown="Default" w457 {
              tunnel: w459 -> [_ w465]
              tunnel: w458 -> [_ w464]
              frame "Test" {
              }
              frame Default {
                n321 = local read "Graph Number"() -> (w460:i32)
                n322 = Format Into String("POLAR_XY" ("input 1"), w464, w460, 0 ("input 2")) -> (resulting string=w463:string)  [unwired: 3 in, 1 out]
                n323 = Enqueue Element(queue=w465, element=w463) -> ()  [unwired: 1 in, 4 out]
              }
            }
          }
        }
      }
      event Shortcut Menu Activation? {
        n324 = event-data() -> ("MenuRef"=w468:refnum<k9>, "Coords"=w466:T14)  [unwired: 6 out]
        n325 = local read "LegendShow"() -> (w469:bool)
        n326 = case shown="True" w469 {
          selector: w469 -> [_ w474]
          tunnel: w468 -> [_ w481]
          tunnel: w467 -> [_ w480]
          tunnel: w466 -> [_ w478]
          frame False {
          }
          frame True {
            n327 = invoke on="Legend" class="MCListbox (strict)" method="Point To Row Column"("Point"=w478) -> ("CellPosition"=w477:T11)  [unwired: 6 in, 6 out]
            n328 = local read "TotalPlot"() -> (w479:u32)
            n329 = control-ref of="Legend"() -> (w472:refnum<vi>)
            n330 = Unbundle By Name(w477) -> ("Row"=w471:i32)
            n331 = local read "LegendVScrollShow"() -> (w470:bool)
            n332 = Less?(x=w471, y=w479) -> (x < y?=w484:bool)
            n333 = Greater?(x=w479, y=u32 0) -> (0:w485:bool)
            n334 = call "CRYGet Selected Data in Legend.vi"("Right Clicked Row"=w471, "Legend Ref"=w472) -> ("Selected Rows"=w473:i32[])  [unwired: 9 in]
            n335 = local write "OldRow"(w471) -> ()
            n336 = local write "SelectedRow"(w473) -> ()
            n337 = property on="Legend" class="MCListbox (strict)"("Value"=w473) -> ()  [unwired: 2 in, 2 out]
            n338 = Bundle By Name(cluster=w480, "LegendShow"=w474, "CellClick"=w484, "Total Number"=w485, "LegendVScrollShow"=w470) -> (w476:T2)
            n339 = control-ref of="This VI"() -> (w475:refnum<vi>)
            n340 = call "CRYGraph Window Menu.vi"("pGraph VI"=w475, "Flag Cluster"=w476, "Type"="LEGEND", "Runtime Menu Ref In"=w481) -> ()  [unwired: 1 in, 7 out]
          }
        }
        n341 = event-data() -> ()  [unwired: 2 in, 1 out]
      }
      event Shortcut Menu Selection (User) {
        n342 = event-data() -> ("ItemTag"=w489:string)  [unwired: 1 out]
        n343 = local read "Graph Number"() -> (w491:i32)
        n344 = case shown="\"DA_LEG_REMOVEALL\"" w489 {
          selector: w489 -> [_ _ _ _ _ _ w527]
          tunnel: w488 -> [_ _ _ _ _ _ _]
          tunnel: w491 -> [_ _ _ _ _ _ _]
          tunnel: w487 -> [_ _ _ _ _ _ _]
          tunnel: [FALSE ("Value (Signaling)") FALSE ("Value (Signaling)") TRUE ("Value (Signaling)") TRUE ("Value (Signaling)") TRUE ("Value (Signaling)") TRUE ("Value (Signaling)") FALSE ("Value (Signaling)")] -> w486
          frame Default {
          }
          frame "DA_LEG_HIDE_1" {
            n345 = control-ref of="This VI"() -> (w496:refnum<vi>)
            n346 = call "CRYData View Legend InsDel.vi"("sOption"="Polar_XY_Legend", "Graph VI Ref"=w496, "sAction"="DA_LEG_HIDE" ("input 2")) -> ()  [unwired: 1 in, 8 out]
          }
          frame "DA_LEG_REMOVE" {
            n347 = property on="RemoveSome" class="Bool (strict)"("Val(Sgnl)"=TRUE ("Value (Signaling)")) -> ()  [unwired: 2 in, 2 out]
          }
          frame "DA_LEG_REMOVEALL" {
            n348 = property on="RemoveAll" class="Bool (strict)"("Val(Sgnl)"=TRUE ("Value (Signaling)")) -> ()  [unwired: 2 in, 2 out]
          }
          frame "DA_LEG_INVERT" {
            n349 = local read "TotalPlot"() -> (w504:u32)
            n350 = for {
              N: w504 -> [_]
              tunnel: [w506] -> w505
              i -> [w508]
              w510 = 38
              w512 = 37
              n351 = property on="Legend" class="MCListbox (strict)"() -> ("ItemSyms"=w514:i32[])  [unwired: 2 in, 2 out]
              n352 = Index Array(array=w514, index=w508) -> (element=w513:i32)
              n353 = To Unsigned Long Integer(number=w508) -> (unsigned 32bit integer=w507:u32)
              n354 = Equal?(x=w513, y=w512) -> (x = y?=w509:bool)
              n355 = Equal?(x=w513, y=w510) -> (x = y?=w511:bool)
              n356 = Select(t=w512, s=w511, f=w510) -> (s? t:f=w515:i32)
              n357 = Replace Array Subset(array=w514, new element=w515, index=w508) -> (w516:i32[])
              n358 = property on="XY Graph" class="XYGraph (strict)"("Active Plot"=w507, "Plot.Visible?"=w509) -> ()  [unwired: 2 in, 2 out]
              n359 = property on="Legend" class="MCListbox (strict)"("ItemSyms"=w516) -> (error out=w506:errorcluster)  [unwired: 2 in, 1 out]
            }
            n360 = property on="AxisChange" class="Bool (strict)"(error in=w505, "Val(Sgnl)"=TRUE ("Value (Signaling)")) -> ()  [unwired: 1 in, 2 out]
          }
          frame "DA_LEG_SHOWALL" {
            n361 = local read "TotalPlot"() -> (w521:u32)
            n362 = for {
              N: w521 -> [_]
              tunnel: [38] -> w518 mode=indexing
              i -> [w525]
              n363 = To Unsigned Long Integer(number=w525) -> (unsigned 32bit integer=w524:u32)
              n364 = property on="XY Graph" class="XYGraph (strict)"("Active Plot"=w524, "Plot.Visible?"=TRUE ("Plot.Visible")) -> ()  [unwired: 2 in, 2 out]
            }
            n365 = property on="Legend" class="MCListbox (strict)"("ItemSyms"=w518) -> (error out=w519:errorcluster)  [unwired: 2 in, 1 out]
            n366 = property on="AxisChange" class="Bool (strict)"(error in=w519, "Val(Sgnl)"=TRUE ("Value (Signaling)")) -> ()  [unwired: 1 in, 2 out]
          }
          frame "DA_LEG_VSCROLL_HIDE", "DA_LEG_VSCROLL_VIEW" {
            n367 = Equal?(x="DA_LEG_VSCROLL_VIEW" ("y"), y=w527) -> (x = y?=w526:bool)
            n368 = property on="LegendVScrollShow" class="Bool (strict)"("Val(Sgnl)"=w526) -> ()  [unwired: 2 in, 2 out]
          }
        }
        n369 = call "CRYPreUpdate Sequence.vi"("EventName"="CurLibUpdate") -> ()  [unwired: 15 in]
        n370 = case shown="True" w486 {
          frame False {
          }
          frame True {
            n371 = property on="XYCursor" class="Str"("Val(Sgnl)"="NamePlot" ("Value (Signaling)")) -> ()  [unwired: 2 in, 2 out]
          }
        }
      }
      event "Frequency": Mouse Down {
        n372 = event-data() -> ("CtlRef"=w534:refnum<vi>, "Coords"=w535:T14, "Button"=w536:u16)  [unwired: 6 out]
        n373 = local read "TotalPlotPolar"() -> (w533:u32)
        n374 = call "CRYData View Legend Plot OnOff.vi"("TotalPlot"=w533, "Button Info"=w536, "Mouse Point"=w535, "MCListbox Ref In"=w534) -> ("Active Row"=w530:i32, "Visible?"=w531:bool, "Click State"=w532:bool)  [unwired: 5 out]
        n375 = case shown="True" w532 {
          tunnel: w531 -> [_ w541]
          tunnel: w530 -> [_ w540]
          frame False {
          }
          frame True {
            n376 = local read "Polar Property"() -> (w539:T1)
            n377 = Unbundle By Name(w539) -> ("Discrete/Rannge"=w538:u16)
            n378 = control-ref of="This VI"() -> (w537:refnum<vi>)
            n379 = call "CRYPlot Polar Graph.vi"("pGraph VI In"=w537, "sOption"="Replot") -> ()  [unwired: 6 in, 4 out]
            n380 = case shown="0, Default" w538 {
              tunnel: w541 -> [w544 _]
              tunnel: w540 -> [w543 _]
              frame 0, Default {
                n381 = property on="XY Graph" class="XYGraph (strict)"("Active Cursor"=w543, "Cursor.Visible"=w544) -> ()  [unwired: 2 in, 2 out]
              }
              frame 1 {
              }
            }
          }
        }
      }
      event "Frequency": Mouse Move {
        n382 = event-data() -> ("Coords"=w552:T14)  [unwired: 5 out]
        n383 = control-ref of="Frequency"() -> (w551:refnum<vi>)
        n384 = local read "TotalPlotPolar"() -> (w550:u32)
        n385 = call "CRYData View Legend Mouse Move.vi"("TotalPlot"=w550, "Mouse Point"=w552, "MCListbox Ref In"=w551) -> ("CellSize"=w546:T7, "Position"=w547:T15, "Selected Row"=w548:i32, "Move State"=w549:bool, "CellBG"=w545:u32)  [unwired: 1 in, 3 out]
        n386 = case shown="True" w549 {
          tunnel: w548 -> [_ w558]
          tunnel: w547 -> [_ w556]
          tunnel: w546 -> [_ w555]
          tunnel: w545 -> [_ w554]
          frame False {
            n387 = property on="ColorBoxPolar" class="ColBox"("Visible"=FALSE) -> ()  [unwired: 2 in, 2 out]
          }
          frame True {
            n388 = local write "OldRowPolar"(w558) -> ()
            n389 = property on="ColorBoxPolar" class="ColBox"("Position"=w556, "Color Area Size"=w555, "Value"=w554) -> ()  [unwired: 2 in, 2 out]
            n390 = property on="ColorBoxPolar" class="ColBox"("Visible"=TRUE) -> ()  [unwired: 2 in, 2 out]
          }
        }
      }
      event "FrequencyVScrollShow": Value Change {
        w569 = T13 {"Left"=0, "Top"=0, "Right"=0, "Bottom"=0}  # input cluster
        n391 = event-data() -> ("NewVal"=w570:bool)  [unwired: 6 out]
        n392 = property on="Frequency" class="MCListbox (strict)"("VScrollVis"=w570) -> ()  [unwired: 2 in, 2 out]
        n393 = control-ref of="PaneFrequency"() -> (w559:refnum<vi>)
        n394 = property class="Pane"(reference=w559) -> ("Left"=w568:i32, "Top"=w565:i32, "Width"=w567:u32, "Height"=w564:u32)  [unwired: 1 in, 2 out]
        n395 = Add(x=w568, y=w567) -> (x+y=w566:u32)
        n396 = Add(x=w565, y=w564) -> (x+y=w563:u32)
        n397 = Bundle By Name(cluster=w569, "Left"=w568, "Top"=w565, "Right"=w566, "Bottom"=w563) -> (w562:T13)
        n398 = local read "FrequencyVScrollShow"() -> (w561:bool)
        n399 = control-ref of="Frequency"() -> (w560:refnum<vi>)
        n400 = call "CRYLegend Resize in Graph Window.vi"("VScrollShow"=w561, "Pane Ref"=w559, "input cluster"=w562, "Legend"=w560) -> ()  [unwired: 8 out]
      }
      event "ColorBoxPolar": Value Change {
        # "Graph Color Changing"
        n401 = event-data() -> ("NewVal"=w573:u32)  [unwired: 6 out]
        n402 = flat-sequence {
          tunnel: w573 -> [w577]
          tunnel: [w575] -> w572
          tunnel: [w574] -> w571
          tunnel: w572 -> [w592]
          tunnel: w571 -> [w591]
          frame #0 {
            n403 = local read "Polar Property"() -> (w576:T1)
            n404 = property on="Frequency" class="MCListbox (strict)"("CellBG"=w577) -> ()  [unwired: 2 in, 2 out]
            n405 = Unbundle By Name(w576) -> ("Discrete/Rannge"=w575:u16)
            n406 = case shown="0, Default" w575 {
              tunnel: w577 -> [w578 w584]
              tunnel: w576 -> [w579 w585]
              tunnel: [w578 w584] -> w574
              frame 0, Default {
                n407 = local read "OldRowPolar"() -> (w581:i32)
                n408 = Unbundle By Name(w579) -> ("CurColors"=w582:u32[])
                n409 = Replace Array Subset(array=w582, new element=w578, index=w581) -> (w580:u32[])
                n410 = Bundle By Name(cluster=w579, "CurColors"=w580) -> (w583:T1)
                n411 = local write "Polar Property"(w583) -> ()
              }
              frame 1 {
                n412 = Unbundle By Name(w585) -> ("CurColors_Range"=w588:u32[])
                n413 = local read "OldRowPolar"() -> (w587:i32)
                n414 = Replace Array Subset(array=w588, new element=w584, index=w587) -> (w586:u32[])
                n415 = Bundle By Name(cluster=w585, "CurColors_Range"=w586) -> (w589:T1)
                n416 = local write "Polar Property"(w589) -> ()
              }
            }
          }
          frame #1 {
            n417 = property on="ColorBoxPolar" class="ColBox"("Visible"=FALSE) -> ()  [unwired: 2 in, 2 out]
            n418 = case shown="0, Default" w592 {
              tunnel: w591 -> [w595 _]
              frame 0, Default {
                n419 = local read "OldRowPolar"() -> (w596:i32)
                n420 = property on="XY Graph" class="XYGraph (strict)"("Active Cursor"=w596, "Cursor.Cursor Color"=w595) -> ()  [unwired: 2 in, 2 out]
              }
              frame 1 {
              }
            }
            n421 = control-ref of="This VI"() -> (w590:refnum<vi>)
            n422 = call "CRYPlot Polar Graph.vi"("pGraph VI In"=w590, "sOption"="Replot") -> ()  [unwired: 6 in, 4 out]
          }
        }
      }
      event "ColorBoxPolar": Mouse Down {
        n423 = event-data() -> ()  [unwired: 9 out]
        n424 = local read "OldRowPolar"() -> (w600:i32)
        n425 = Bundle By Name(cluster=T11 {"Row"=0, "Column"=0} ("Active Cell:Active Cell"), "Row"=w600, "Column"=1) -> (w597:T11)
        n426 = property on="Frequency" class="MCListbox (strict)"("ActiveCell"=w597) -> ()  [unwired: 2 in, 2 out]
      }
      event "Legend": Mouse Down {
        n427 = event-data() -> ("CtlRef"=w603:refnum<vi>, "Coords"=w601:T14, "Button"=w602:u16)  [unwired: 6 out]
        n428 = local read "TotalPlot"() -> (w606:u32)
        n429 = call "CRYData View Legend Plot OnOff.vi"("TotalPlot"=w606, "Button Info"=w602, "Mouse Point"=w601, "MCListbox Ref In"=w603) -> ("Active Row"=w607:i32, "Visible?"=w605:bool, "Click State"=w604:bool)  [unwired: 5 out]
        n430 = case shown="True" w604 {
          tunnel: w605 -> [_ w614]
          tunnel: w607 -> [_ w615]
          frame False {
          }
          frame True {
            w610 = u8 0 ("Y Scale.Scale Fit")
            n431 = property on="XY Graph" class="XYGraph (strict)"("XScale.ScaleFit"=w610) -> ()  [unwired: 2 in, 2 out]
            n432 = property on="XY Graph" class="XYGraph (strict)"("XScale.ScaleFit"=w610) -> (error out=w611:errorcluster)  [unwired: 2 in, 1 out]
            n433 = property on="AxisChange" class="Bool (strict)"("Val(Sgnl)"=TRUE ("Value (Signaling)")) -> ()  [unwired: 2 in, 2 out]
            n434 = To Unsigned Long Integer(number=w615) -> (unsigned 32bit integer=w613:u32)
            n435 = property on="XY Graph" class="XYGraph (strict)"(error in=w611, "Active Plot"=w613, "Plot.Visible?"=w614) -> (error out=w608:errorcluster)  [unwired: 1 in, 1 out]
            n436 = property on="XYCursor" class="Str"(error in=w608, "Val(Sgnl)"="NamePlot" ("Value (Signaling)")) -> ()  [unwired: 1 in, 2 out]
          }
        }
      }
      event "Legend": Mouse Move {
        n437 = event-data() -> ("CtlRef"=w617:refnum<vi>, "Coords"=w616:T14)  [unwired: 4 out]
        n438 = local read "TotalPlot"() -> (w618:u32)
        n439 = call "CRYData View Legend Mouse Move.vi"("TotalPlot"=w618, "Mouse Point"=w616, "MCListbox Ref In"=w617) -> ("CellSize"=w620:T7, "Position"=w621:T15, "Selected Row"=w622:i32, "Move State"=w623:bool, "CellBG"=w619:u32)  [unwired: 1 in, 3 out]
        n440 = case shown="True" w623 {
          tunnel: w619 -> [_ w629]
          tunnel: w620 -> [_ w628]
          tunnel: w621 -> [_ w627]
          tunnel: w622 -> [_ w626]
          frame False {
            n441 = property on="ColorBox" class="ColBox"("Visible"=FALSE) -> ()  [unwired: 2 in, 2 out]
          }
          frame True {
            n442 = local write "OldRow"(w626) -> ()
            n443 = property on="ColorBox" class="ColBox"("Position"=w627, "Color Area Size"=w628, "Value"=w629, "Visible"=TRUE) -> ()  [unwired: 2 in, 2 out]
          }
        }
      }
      event "Legend": Value Change {
        n444 = event-data() -> ("NewVal"=w630:i32[])  [unwired: 6 out]
        n445 = local read "Test"() -> (w631:string)
        n446 = case shown="Default" w631 {
          tunnel: w630 -> [w633 _]
          frame Default {
            n447 = local read "GraphType"() -> (w635:string)
            n448 = control-ref of="Legend"() -> (w634:refnum<vi>)
            n449 = call "CRYData View Legend Manipulate.vi"("sAction"="GetViewNumbyLegNum", "nData"=w633, "sData"=w635, "Legend Ref"=w634) -> ("nData Out"=w636:i32[])  [unwired: 6 in, 1 out]
            n450 = call "CRYGet Graph Name From Graph Type.vi"("Graph Type"=w635) -> ("Type"=w638:enum16{"Curves", "Values", "Results", "WFM"})  [unwired: 9 in, 1 out]
            n451 = call "CRYTree Global Manipulate.vi"("Type In"=w638) -> ("Tree/Curve Tree"=w637:refnum<vi>)  [unwired: 7 in, 3 out]
            n452 = call "CRYTree Manuplate.vi"("sAction"="SetActiveNumbers", "nData"=w636, "Tree in"=w637) -> ("Tree Out"=w632:refnum<vi>)  [unwired: 5 in, 3 out]
            n453 = flat-sequence {
              tunnel: w632 -> [_]
              frame #0 {
                n454 = call "CRYUpdate Buttons.vi"() -> ()  [unwired: 12 in]
              }
            }
          }
          frame "Test" {
          }
        }
      }
      event "LegendVScrollShow": Value Change {
        w652 = T13 {"Left"=0, "Top"=0, "Right"=0, "Bottom"=0}  # input cluster
        n455 = event-data() -> ("NewVal"=w644:bool)  [unwired: 6 out]
        n456 = property on="Legend" class="MCListbox (strict)"("VScrollVis"=w644) -> ()  [unwired: 2 in, 2 out]
        n457 = control-ref of="PaneLegend"() -> (w643:refnum<vi>)
        n458 = property class="Pane"(reference=w643) -> ("Left"=w651:i32, "Top"=w648:i32, "Width"=w650:u32, "Height"=w647:u32)  [unwired: 1 in, 2 out]
        n459 = Add(x=w651, y=w650) -> (x+y=w649:u32)
        n460 = Add(x=w648, y=w647) -> (x+y=w646:u32)
        n461 = Bundle By Name(cluster=w652, "Left"=w651, "Top"=w648, "Right"=w649, "Bottom"=w646) -> (w645:T13)
        n462 = local read "LegendVScrollShow"() -> (w641:bool)
        n463 = control-ref of="Legend"() -> (w642:refnum<vi>)
        n464 = call "CRYLegend Resize in Graph Window.vi"("VScrollShow"=w641, "Pane Ref"=w643, "input cluster"=w645, "Legend"=w642) -> ()  [unwired: 8 out]
      }
      event "ColorBox": Value Change {
        # "Graph Color Changing"
        n465 = event-data() -> ("NewVal"=w653:u32)  [unwired: 6 out]
        n466 = local read "OldRow"() -> (w654:i32)
        n467 = local read "Event Name"() -> (w656:string)
        n468 = flat-sequence {
          tunnel: [w665] -> w657
          tunnel: w653 -> [w665]
          tunnel: w654 -> [w664]
          tunnel: w657 -> [w666]
          frame #0 {
            n469 = To Unsigned Long Integer(number=w664) -> (unsigned 32bit integer=w663:u32)
            n470 = property on="Legend" class="MCListbox (strict)"("CellBG"=w665) -> ()  [unwired: 2 in, 2 out]
            n471 = property on="XY Graph" class="XYGraph (strict)"("Active Plot"=w663) -> ()  [unwired: 2 in, 2 out]
          }
          frame #1 {
            n472 = property on="XY Graph" class="XYGraph (strict)"("Plot.Plot Color"=w666) -> ()  [unwired: 2 in, 2 out]
            n473 = property on="ColorBox" class="ColBox"("Visible"=FALSE) -> ()  [unwired: 2 in, 2 out]
          }
        }
        n474 = call "CRYPreUpdate Sequence.vi"("EventName"="CurLibUpdate") -> ()  [unwired: 15 in]
        n475 = case shown="Default" w656 {
          tunnel: w654 -> [_ w661]
          tunnel: w653 -> [_ w660]
          frame "ViewReport" {
          }
          frame Default {
            n476 = control-ref of="Legend"() -> (w659:refnum<vi>)
            n477 = call "CRYSet Plot Settings.vi"("sAction"="Color", "Color"=w660, "Row"=w661, "Legend Refnum"=w659, "Type"=enum16{"Curves", "Values", "Results", "WFM"}."Curves") -> ()  [unwired: 2 in, 5 out]
          }
        }
      }
      event "ColorBox": Mouse Down {
        n478 = event-data() -> ()  [unwired: 9 out]
        n479 = local read "OldRow"() -> (w668:i32)
        n480 = Bundle By Name(cluster=T11 {"Row"=0, "Column"=0} ("Active Cell:Active Cell"), "Row"=w668, "Column"=1) -> (w671:T11)
        n481 = property on="Legend" class="MCListbox (strict)"("ActiveCell"=w671) -> ()  [unwired: 2 in, 2 out]
      }
      event "RemoveSome": Value Change {
        n482 = event-data() -> ()  [unwired: 7 out]
        n483 = flat-sequence {
          tunnel: [w675] -> w673
          tunnel: [w680] -> w672
          tunnel: w673 -> [w705]
          tunnel: w672 -> [w704]
          frame #0 {
            n484 = local read "SelectedRow"() -> (w679:i32[])
            n485 = control-ref of="Legend"() -> (w677:refnum<vi>)
            n486 = Reverse 1D Array(array=w679) -> (reversed array=w675:i32[])
            n487 = local read "GraphType"() -> (w674:string)
            n488 = for {
              shift-right: [w685] -> w680
              shift-left: _ -> [w684]
              tunnel: w675 -> [w683] mode=indexing
              n489 = local read "TotalPlot"() -> (w689:u32)
              n490 = Decrement(x=w689) -> (x-1=w688:u32)
              n491 = Increment(x=w683) -> (x+1=w686:i32)
              n492 = Subtract(x=w688, y=w683) -> (x-y=w687:u32)
              n493 = for {
                N: w687 -> [_]
                tunnel: w686 -> [w696]
                shift-right: [w692] -> w685
                shift-left: w684 -> [w691]
                i -> [w695]
                n494 = Add(x=w696, y=w695) -> (x+y=w693:i32)
                n495 = Decrement(x=w693) -> (x-1=w694:i32)
                n496 = property on="XY Graph" class="XYGraph (strict)"(error in=w691, "Active Plot"=w693) -> (error out=w690:errorcluster, "Plot.Plot Color"=w703:u32, "Plot.Fill/Pt. Color"=w702:u32, "Plot.Fill To"=w701:i16, "Plot.Line Style"=w700:u8, "Plot.Line Width"=w699:u8, "Plot.Point Style"=w698:u8, "Plot.Plot Interpolation"=w697:u8)  [unwired: 1 in, 1 out]
                n497 = property on="XY Graph" class="XYGraph (strict)"(error in=w690, "Active Plot"=w694, "Plot.Plot Color"=w703, "Plot.Fill/Pt. Color"=w702, "Plot.Fill To"=w701, "Plot.Line Style"=w700, "Plot.Line Width"=w699, "Plot.Point Style"=w698, "Plot.Plot Interpolation"=w697) -> (error out=w692:errorcluster)  [unwired: 1 in, 1 out]
              }
              n498 = local write "TotalPlot"(w688) -> ()
            }
            n499 = call "CRYData View Legend Manipulate.vi"("sAction"="GetGlobalNumbyLegNum", "nData"=w675, "sData"=w674, "Legend Ref"=w677) -> ("nData Out"=w676:i32[])  [unwired: 6 in, 1 out]
            n500 = control-ref of="This VI"() -> (w681:refnum<vi>)
            n501 = call "CRYSymbol Conversion.vi"("pGraph VI"=w681, "nDatas"=w676, "sActin"="LEGEND_REMOVE") -> ()  [unwired: 9 in]
          }
          frame #1 {
            n502 = for {
              tunnel: w705 -> [w706] mode=indexing
              n503 = control-ref of="Legend"() -> (w709:refnum<vi>)
              n504 = local read "XY Graph"() -> (w708:cluster{"XY Graph":cluster{dbl, dbl}[]}[])
              n505 = Delete From Array(array=w708, index=w706) -> (array with subset deleted=w707:cluster{"XY Graph":cluster{dbl, dbl}[]}[])  [unwired: 1 in, 1 out]
              n506 = call "CRYData View Legend Item Delete.vi"("RowNumber"=w706, "Legend MultiListbox In"=w709) -> ()  [unwired: 10 out]
              n507 = local write "XY Graph"(w707) -> ()
            }
            n508 = case shown="No Error" w704 {
              frame No Error {
              }
              frame Error {
              }
            }
          }
          frame #2 {
            n509 = local read "TotalPlot"() -> (w712:u32)
            n510 = case shown="1, Default" w712 {
              selector: w712 -> [_ w716]
              frame 0 {
                n511 = property on="RemoveAll" class="Bool (strict)"("Val(Sgnl)"=TRUE ("Value (Signaling)")) -> ()  [unwired: 2 in, 2 out]
              }
              frame 1, Default {
                n512 = for {
                  N: w716 -> [_]
                  tunnel: [w717] -> w714
                  i -> [w720]
                  n513 = property on="Legend" class="MCListbox (strict)"() -> ("ItemSyms"=w723:i32[])  [unwired: 2 in, 2 out]
                  n514 = Bundle By Name(cluster=T11 {"Row"=0, "Column"=0} ("Active Cell:Active Cell"), "Row"=w720, "Column"=1) -> (w724:T11)
                  n515 = Index Array(array=w723, index=w720) -> (element=w721:i32)
                  n516 = property on="Legend" class="MCListbox (strict)"("ActiveCell"=w724) -> ("CellBG"=w719:u32)  [unwired: 2 in, 2 out]
                  n517 = Equal?(x=w721, y=38) -> (x = y?=w718:bool)
                  n518 = property on="XY Graph" class="XYGraph (strict)"("Active Plot"=w720, "Plot.Plot Color"=w719, "Plot.Fill/Pt. Color"=w719, "Plot.Visible?"=w718) -> (error out=w717:errorcluster)  [unwired: 2 in, 1 out]
                }
                n519 = property on="AxisChange" class="Bool (strict)"("Val(Sgnl)"=TRUE ("Value (Signaling)")) -> ()  [unwired: 2 in, 2 out]
                n520 = case shown="No Error" w714 {
                  frame No Error {
                  }
                  frame Error {
                  }
                }
              }
            }
            n521 = control-ref of="This VI"() -> (w710:refnum<vi>)
            n522 = call "CRYPlot Polar Graph.vi"("pGraph VI In"=w710, "sOption"="Replot") -> ()  [unwired: 6 in, 4 out]
          }
        }
      }
      event "RemoveAll": Value Change {
        w734 = i16 0 ("left")
        w746 = 0 ("Active X Scale")
        w748 = "" ("X Scale.Name Label.Text")
        n523 = event-data() -> ()  [unwired: 7 out]
        n524 = property on="Polar Plot" class="Pict"() -> ("Draw Area Size"=w727:T7)  [unwired: 2 in, 2 out]
        n525 = local read "Polar Property"() -> (w738:T1)
        n526 = Unbundle By Name(w727) -> ("Width"=w735:u32, "Height"=w736:u32)
        n527 = Bundle By Name(cluster=T10 {"left"=0, "top"=0, "right"=0, "bottom"=0} ("rect"), "left"=w734, "top"=w734, "right"=w735, "bottom"=w736) -> (w730:T10)
        n528 = Unbundle By Name(w738) -> ("BackgroundColor"=w728:u32, "polar attributes"=w737:T8)
        n529 = Bundle By Name(cluster=w737, "maximum"=1.0, "minimum"=-1.0) -> (w741:T8)
        n530 = call <vilib>:"Draw Rect.vi"("picture"=picture data[5B] ("Value"), "rect"=w730, "fill?(F)"=TRUE, "color(black)"=w728) -> ("new picture"=w729:picture)  [unwired: 5 in]
        n531 = call <vilib>:"Polar Plot.vi"("polar attributes"=w741, "dimensions (w,h)"=w727, "data array [mag, phase (deg)]"=cluster{"magnitude":dbl, "phase":dbl}[] [], "picture"=w729) -> ("new picture"=w739:picture)  [unwired: 7 out]
        n532 = property on="Polar Plot" class="Pict"("Value"=w739) -> ()  [unwired: 2 in, 2 out]
        n533 = flat-sequence {
          frame #0 {
            n534 = control-ref of="This VI"() -> (w755:refnum<vi>)
            n535 = Build Array(-1 ("nData")) -> (w756:i32[])
            n536 = call "CRYSymbol Conversion.vi"("pGraph VI"=w755, "nDatas"=w756, "sActin"="LEGEND_REMOVE") -> ()  [unwired: 9 in]
          }
          frame #1 {
            n537 = control-ref of="Legend"() -> (w759:refnum<vi>)
            n538 = call "CRYData View Legend Item Delete.vi"("RowNumber"=-1, "Legend MultiListbox In"=w759) -> ()  [unwired: 10 out]
          }
        }
        n539 = local write "TotalPlot"(u32 0 ("TotalPlot")) -> ()
        n540 = local write "OldRow"(-1 ("OldRow 2")) -> ()
        n541 = flat-sequence {
          frame #0 {
            n542 = local write "XY Graph"(cluster{"XY Graph":cluster{dbl, dbl}[]}[] [] ("XY Graph")) -> ()
          }
          frame #1 {
            n543 = property on="Repaint Watermark" class="DigNum (strict)"("Val(Sgnl)"=-1 ("Value (Signaling)")) -> ()  [unwired: 2 in, 2 out]
          }
        }
        n544 = property on="XY Graph" class="XYGraph (strict)"("ActXScl"=w746, "XScale.NameLbl.Text"=w748, "ActYScl"=w746, "YScale.NameLbl.Text"=w748, "ActYScl"=1 ("Active Y Scale"), "YScale.NameLbl.Text"=w748, "YScale.Visible"=FALSE ("Y Scale.Visible")) -> ()  [unwired: 2 in, 2 out]
        n545 = property on="XY Graph" class="XYGraph (strict)"("ActXScl"=0 ("Active X Scale"), "XScale.ScaleFit"=u8 2 ("X Scale.Scale Fit")) -> ()  [unwired: 2 in, 2 out]
      }
      event "AxisChange": Value Change {
        w779 = enum16{"Curves", "Values", "Results", "WFM"}."Curves" ("Type In")
        n546 = event-data() -> ()  [unwired: 7 out]
        n547 = control-ref of="Legend"() -> (w769:refnum<vi>)
        n548 = call "CRYGet Graph Data in Graph.vi"("Graph Type"="XY", "Legend Refnum"=w769, "Type In"=w779) -> ("Rows"=w767:i32[])  [unwired: 4 in, 4 out]
        n549 = property on="Legend" class="MCListbox (strict)"() -> ("ItemSyms"=w768:i32[])  [unwired: 2 in, 2 out]
        n550 = for {
          tunnel: w768 -> [w805] mode=indexing
          shift-right: [w804] -> w776
          shift-left: i32[] [] -> [w803]
          tunnel: w767 -> [w802] mode=indexing
          shift-right: [w799] -> w778
          shift-left: i32[] [] -> [w798]
          i -> [w800]
          n551 = Equal?(x=38, y=w805) -> (x = y?=w801:bool)
          n552 = case shown="True" w801 {
            tunnel: [w808 w814] -> w804
            tunnel: w803 -> [w808 w813]
            tunnel: w802 -> [_ w812]
            tunnel: w800 -> [_ w811]
            tunnel: [w807 w810] -> w799
            tunnel: w798 -> [w807 w809]
            frame False {
            }
            frame True {
              n553 = Insert Into Array(array=w809, new element=w811) -> (w810:i32[])  [unwired: 1 in]
              n554 = Insert Into Array(array=w813, new element=w812) -> (w814:i32[])  [unwired: 1 in]
            }
          }
        }
        n555 = call "CRYGet Legend Name.vi"("MCListbox Refnum"=w769) -> ("Names Out"=w770:string[])  [unwired: 10 in]
        n556 = control-ref of="This VI"() -> (w761:refnum<vi>)
        n557 = call "CRYGet Two Units Rows.vi"("pGraph VI In"=w761, "Old Rows In"=w776, "Type"=w779) -> ("Unit2"=w765:string, "Unit1"=w775:string, "Two Units"=w764:i32)  [unwired: 2 in, 4 out]
        n558 = for {
          tunnel: w770 -> [w787]
          tunnel: w778 -> [w788] mode=indexing
          tunnel: [w784] -> w772 mode=indexing
          tunnel: [w783] -> w773 mode=indexing
          tunnel: [w782] -> w771
          tunnel: w779 -> [w781]
          n559 = Index Array(array=w787, index=w788) -> (element=w786:string)
          n560 = call "CRYGet Curve Library Data.vi"("Type"=w781, "Data Name"=w786) -> ("Curve"=w785:T16)  [unwired: 4 out]
          n561 = Unbundle By Name(w785) -> ("Y unit"=w784:string, "Z unit"=w783:string, "X unit"=w782:string)
        }
        n562 = local read "MagnitudeShow"() -> (w762:bool)
        n563 = Select(t=w772, s=w762, f=w773) -> (s? t:f=w774:string[])
        n564 = case shown="2, Default" w764 {
          selector: w764 -> [w815 w823 w828]
          tunnel: w775 -> [w818 _ w833]
          tunnel: w765 -> [w820 _ _]
          tunnel: w771 -> [w816 _ w831]
          tunnel: [w815 w823 w828] -> w780
          frame 2, Default {
            n565 = property on="XY Graph" class="XYGraph (strict)"("ActXScl"=0 ("Active X Scale"), "XScale.NameLbl.Text"=w816, "ActYScl"=0 ("Active Y Scale"), "YScale.NameLbl.Text"=w818, "ActYScl"=1 ("Active Y Scale"), "YScale.Visible"=TRUE ("Y Scale.Visible"), "YScale.NameLbl.Text"=w820) -> ()  [unwired: 2 in, 2 out]
          }
          frame 0 {
            w827 = 0 ("Active X Scale")
            w825 = "" ("X Scale.Name Label.Text")
            n566 = property on="XY Graph" class="XYGraph (strict)"("ActXScl"=w827, "XScale.NameLbl.Text"=w825, "ActYScl"=w827, "YScale.NameLbl.Text"=w825, "ActYScl"=1 ("Active Y Scale"), "YScale.NameLbl.Text"=w825, "YScale.Visible"=FALSE ("Y Scale.Visible")) -> ()  [unwired: 2 in, 2 out]
          }
          frame 1 {
            n567 = property on="XY Graph" class="XYGraph (strict)"("ActXScl"=0 ("Active X Scale"), "XScale.NameLbl.Text"=w831, "ActYScl"=0 ("Active Y Scale"), "YScale.NameLbl.Text"=w833, "ActYScl"=1 ("Active Y Scale"), "YScale.Visible"=FALSE ("Y Scale.Visible")) -> ()  [unwired: 2 in, 2 out]
          }
        }
        n568 = for {
          tunnel: w778 -> [w797] mode=indexing
          tunnel: w774 -> [w795] mode=indexing
          tunnel: w775 -> [w796]
          shift-right: [w790] -> w760
          shift-left: _ -> [w789]
          n569 = Equal?(x=w796, y=w795) -> (x = y?=w794:bool)
          n570 = Select(t=u32 0 ("Plot.Y Scale Index"), s=w794, f=u32 1 ("Plot.Y Scale Index")) -> (s? t:f=w791:u32)
          n571 = property on="XY Graph" class="XYGraph (strict)"(error in=w789, "Active Plot"=w797, "Plot.YScaleIdx"=w791) -> (error out=w790:errorcluster)  [unwired: 1 in, 1 out]
        }
        n572 = case shown="No Error" w760 {
          frame No Error {
          }
          frame Error {
          }
        }
        n573 = property on="Repaint Watermark" class="DigNum (strict)"("Val(Sgnl)"=w780) -> ()  [unwired: 2 in, 2 out]
      }
      event "Repaint Watermark": Value Change {
        # "Repaint Watermark: 0-none, 1-Unit 1, 2-Unit 1 & 2, -1: surely replot"
        n574 = event-data() -> ("OldVal"=w835:i32, "NewVal"=w836:i32)  [unwired: 5 out]
        n575 = Equal?(x=-1 ("y"), y=w836) -> (x = y?=w839:bool)
        n576 = case shown="False" w839 {
          tunnel: w835 -> [w843 w858]
          tunnel: [w842 "Replot" ("PropertyTab")] -> w837
          tunnel: w836 -> [w841 _]
          tunnel: [w841 w858] -> w840
          frame False {
            n577 = Not Equal?(x=w843, y=w841) -> (x != y?=w844:bool)
            n578 = case shown="True" w844 {
              tunnel: w843 -> [_ w851]
              tunnel: w841 -> [_ w850]
              tunnel: [_ w845] -> w842
              frame False {
              }
              frame True {
                n579 = Equal To 0?(x=w851) -> (x = 0?=w855:bool)
                n580 = Equal?(x=w850, y=1) -> (x = y?=w856:bool)
                n581 = Equal?(x=w851, y=1) -> (x = y?=w849:bool)
                n582 = Equal To 0?(x=w850) -> (x = 0?=w848:bool)
                n583 = And(x=w849, y=w848) -> (x .and. y?=w847:bool)
                n584 = And(x=w855, y=w856) -> (x .and. y?=w853:bool)
                n585 = Or(x=w853, y=w847) -> (x .or. y?=w846:bool)
                n586 = case shown="False" w846 {
                  tunnel: ["Replot" ("PropertyTab") _] -> w845
                  frame False {
                  }
                  frame True {
                  }
                }
              }
            }
          }
          frame True {
          }
        }
        n587 = local write "Repaint Watermark"(w840) -> ()
        n588 = case shown="\"Replot\"" w837 {
          frame Default {
          }
          frame "Replot" {
            n589 = property on="XY Graph" class="XYGraph (strict)"("PlotImages.Front"=picture data[5B] ("Plot Images:Front")) -> (error out=w864:errorcluster)  [unwired: 2 in, 1 out]
            n590 = local read "Event Name"() -> (w860:string)
            n591 = property on="XY Graph" class="XYGraph (strict)"(error in=w864) -> ("Plot Bounds"=w862:T13)  [unwired: 1 in, 2 out]
            n592 = call "CRYGetWaterMark.vi"("Type"=w860, "Plot Area Bounds"=w862) -> ("WaterMark Image"=w863:picture)  [unwired: 2 in, 7 out]
            n593 = property on="XY Graph" class="XYGraph (strict)"("PlotImages.Front"=w863) -> ()  [unwired: 2 in, 2 out]
          }
        }
      }
      event "OpenProperty": Value Change {
        n594 = event-data() -> ()  [unwired: 7 out]
        n595 = flat-sequence {
          frame #0 {
            n596 = local read "PropertyTab"() -> (w865:string)
            n597 = control-ref of="This VI"() -> (w866:refnum<vi>)
            n598 = call "CRYGraph Property Window Main.vi"("TabName"=w865, "pGraph VI In"=w866) -> ()  [unwired: 1 in, 9 out]
          }
          frame #1 {
            n599 = local write "PropertyTab"("" ("PropertyTab")) -> ()
          }
        }
      }
      event "XYCursor": Value Change {
        n600 = event-data() -> ("CtlRef"=w869:refnum<vi>, "NewVal"=w871:string)  [unwired: 5 out]
        n601 = local read "Polar Property"() -> (w870:T1)
        n602 = property class="Str"(reference=w869, "Value"="") -> ()  [unwired: 1 in, 2 out]
        n603 = case shown="\"Range\"" w871 {
          selector: w871 -> [w872 _ _ _ _ _ _ _ _ _ _ _ _ _]
          tunnel: w870 -> [w873 w941 _ _ w960 w976 w981 w1023 w1042 _ w1077 _ _ _]
          frame Default {
            n604 = Match Pattern(string=w872, regular expression="CurValue") -> (after substring=w875:string, offset past match=w874:i32)  [unwired: 1 in, 2 out]
            n605 = case shown="Default" w874 {
              tunnel: w875 -> [w882 _]
              tunnel: w873 -> [w881 w912]
              tunnel: w872 -> [_ w910]
              frame Default {
                n606 = Unbundle By Name(w881) -> ("CurIndex"=w877:u16, "Discrete/Rannge"=w878:u16, "CurValues"=w879:dbl[])
                n607 = Decimal String To Number(string=w882) -> (number=w880:i32)  [unwired: 2 in, 1 out]
                n608 = case shown="0, Default" w878 {
                  tunnel: w880 -> [w890 w906]
                  tunnel: w879 -> [w889 w907]
                  tunnel: w877 -> [_ w905]
                  frame 0, Default {
                    n609 = Index Array(array=w889, index=w890) -> (element=w884:dbl)
                    n610 = Add(x=w884, y=0.5) -> (x+y=w887:dbl)
                    n611 = Round Toward -Infinity(1:w887) -> (0:w886:dbl)
                    n612 = Format Value(format string="%.0f" ("string"), value (0)=w886) -> (output string=w883:string)  [unwired: 1 in]
                    n613 = property on="XY Graph" class="XYGraph (strict)"("Active Cursor"=w890, "Cursor.Cursor X"=w884, "Cursor.Cursor Name"=w883) -> ()  [unwired: 2 in, 2 out]
                  }
                  frame 1 {
                    n614 = Index Array(array=w907, index=w906) -> (element=w899:dbl)
                    n615 = Add(x=w899, y=0.5) -> (x+y=w902:dbl)
                    n616 = Round Toward -Infinity(1:w902) -> (0:w901:dbl)
                    n617 = Subtract(x=w906, y=w905) -> (x-y=w897:i32)
                    n618 = Format Value(format string="%.0f" ("string"), value (0)=w901) -> (output string=w898:string)  [unwired: 1 in]
                    n619 = property on="XY Graph" class="XYGraph (strict)"("Active Cursor"=w897, "Cursor.Cursor X"=w899, "Cursor.Cursor Name"=w898) -> (error out=w892:errorcluster)  [unwired: 2 in, 1 out]
                    n620 = property on="XY Graph" class="XYGraph (strict)"(error in=w892) -> ("Value"=w895:cluster{"XY Graph":cluster{dbl, dbl}[]}[])  [unwired: 1 in, 2 out]
                    n621 = Array Size(array=w895) -> (size(s)=w894:i32)
                    n622 = Decrement(x=w894) -> (x-1=w893:i32)
                    n623 = Delete From Array(array=w895, index=w893) -> (array with subset deleted=w896:cluster{"XY Graph":cluster{dbl, dbl}[]}[])  [unwired: 1 in, 1 out]
                    n624 = property on="XY Graph" class="XYGraph (strict)"("Value"=w896) -> (error out=w891:errorcluster)  [unwired: 2 in, 1 out]
                    n625 = property on="XYCursor" class="Str"(error in=w891, "Val(Sgnl)"="Fill" ("Value (Signaling)")) -> ()  [unwired: 1 in, 2 out]
                  }
                }
              }
              frame -1 {
                n626 = Match Pattern(string=w910, regular expression="CurColor") -> (after substring=w908:string, offset past match=w909:i32)  [unwired: 1 in, 2 out]
                n627 = case shown="Default" w909 {
                  tunnel: w912 -> [_ w918]
                  tunnel: w908 -> [_ w914]
                  frame -1 {
                  }
                  frame Default {
                    n628 = Unbundle By Name(w918) -> ("CurIndex"=w913:u16, "Discrete/Rannge"=w917:u16, "CurColors"=w915:u32[])
                    n629 = Decimal String To Number(string=w914) -> (number=w916:i32)  [unwired: 2 in, 1 out]
                    n630 = case shown="1" w917 {
                      tunnel: w916 -> [w920 w924]
                      tunnel: w915 -> [w921 w926]
                      tunnel: w913 -> [_ w923]
                      frame 0, Default {
                        n631 = Index Array(array=w921, index=w920) -> (element=w919:u32)
                        n632 = property on="XY Graph" class="XYGraph (strict)"("Active Cursor"=w920, "Cursor.Cursor Color"=w919) -> ()  [unwired: 2 in, 2 out]
                      }
                      frame 1 {
                        n633 = Index Array(array=w926, index=w924) -> (element=w925:u32)
                        n634 = Subtract(x=w924, y=w923) -> (x-y=w922:i32)
                        n635 = property on="XY Graph" class="XYGraph (strict)"("Active Cursor"=w922, "Cursor.Cursor Color"=w925) -> ()  [unwired: 2 in, 2 out]
                      }
                    }
                  }
                }
              }
            }
          }
          frame "Add" {
            n636 = Unbundle By Name(w941) -> ("CurColors"=w928:u32[], "CurValues"=w931:dbl[])
            n637 = property on="XY Graph" class="XYGraph (strict)"("ActYScl"=0 ("Active Y Scale")) -> ("YScale.Increment"=w946:dbl, "YScale.Minimum"=w945:dbl)  [unwired: 2 in, 2 out]
            n638 = Array Size(array=w928) -> (size(s)=w930:i32)
            n639 = Decrement(x=w930) -> (x-1=w929:i32)
            n640 = Subtract(x=w945, y=w946) -> (x-y=w943:dbl)
            n641 = Multiply(x=w946, y=2.0) -> (x*y=w944:dbl)
            n642 = Index Array(array=w931, index=w929) -> (element=w933:dbl)
            n643 = Index Array(array=w928, index=w929) -> (element=w938:u32)
            n644 = Add(x=w933, y=0.5) -> (x+y=w936:dbl)
            n645 = Round Toward -Infinity(1:w936) -> (0:w935:dbl)
            n646 = Format Value(format string="%.0f" ("string"), value (0)=w935) -> (output string=w932:string)  [unwired: 1 in]
            n647 = Bundle By Name(cluster=T12 {"Name"="", "Color"=0, "Style"=2, "Point Style"=0, "Name Visible"=TRUE, "Allow Drag"=TRUE, "Cursor Mode"=0, "Plot"=0, "Index"=0, "Position"={"X"=0.0, "Y"=0.0}, "X Scale"=0, "Y Scale"=0, "Watch Plots"=[], "Watch All Plots"=FALSE, "Plot Area"=0, "Label Offset"={"X"=0.0, "Y"=0.2}} ("new element/subarray"), "Name"=w932, "Color"=w938, "Position.X"=w933, "Position.Y"=w943, "Label Offset.Y"=w944) -> (w950:T12)
            n648 = property on="XY Graph" class="XYGraph (strict)"() -> ("CrsrList"=w942:T5)  [unwired: 2 in, 2 out]
            n649 = Insert Into Array(array=w942, new element=w950) -> (w948:T5)  [unwired: 1 in]
            n650 = property on="XY Graph" class="XYGraph (strict)"("CrsrList"=w948) -> (error out=w939:errorcluster)  [unwired: 2 in, 1 out]
            n651 = property on="XY Graph" class="XYGraph (strict)"(error in=w939, "Active Cursor"=w929, "Cursor.LineWidth"=u8 2 ("Cursor.Line Width")) -> (error out=w927:errorcluster)  [unwired: 1 in, 1 out]
            n652 = case shown="No Error" w927 {
              frame No Error {
              }
              frame Error {
              }
            }
          }
          frame "Delete" {
            n653 = property on="XY Graph" class="XYGraph (strict)"() -> ("CrsrList"=w954:T5)  [unwired: 2 in, 2 out]
            n654 = Array Size(array=w954) -> (size(s)=w953:i32)
            n655 = Decrement(x=w953) -> (x-1=w952:i32)
            n656 = Delete From Array(array=w954, index=w952) -> (array with subset deleted=w955:T5)  [unwired: 1 in, 1 out]
            n657 = property on="XY Graph" class="XYGraph (strict)"("CrsrList"=w955) -> ()  [unwired: 2 in, 2 out]
          }
          frame "DeleteSelf" {
            # "From frequency popup menu, Remove one frequency."
            n658 = property on="XY Graph" class="XYGraph (strict)"() -> ("CrsrList"=w957:T5)  [unwired: 2 in, 2 out]
            n659 = local read "OldRowPolar"() -> (w956:i32)
            n660 = Delete From Array(array=w957, index=w956) -> (array with subset deleted=w958:T5)  [unwired: 1 in, 1 out]
            n661 = property on="XY Graph" class="XYGraph (strict)"("CrsrList"=w958) -> ()  [unwired: 2 in, 2 out]
          }
          frame "DeleteAll" {
            # "From frequency popup menu, Remove all frequency."
            n662 = Unbundle By Name(w960) -> ("Discrete/Rannge"=w963:u16, "CurValues"=w962:dbl[], "CurIndex"=w961:u16)
            n663 = case shown="1" w963 {
              tunnel: w962 -> [_ w967]
              tunnel: w961 -> [_ w965]
              tunnel: w960 -> [_ w969]
              frame 0, Default {
              }
              frame 1 {
                w970 = 0.0 ("new element/subarray")
                n664 = Increment(x=w965) -> (x+1=w964:u16)
                n665 = property on="XY Graph" class="XYGraph (strict)"() -> ("Value"=w973:cluster{"XY Graph":cluster{dbl, dbl}[]}[])  [unwired: 2 in, 2 out]
                n666 = Replace Array Subset(array=w967, new element #1=w970, index #1=w965, new element #2=w970, index #2=w964) -> (w968:dbl[])
                n667 = Array Size(array=w973) -> (size(s)=w972:i32)
                n668 = Decrement(x=w972) -> (x-1=w971:i32)
                n669 = Bundle By Name(cluster=w969, "CurValues"=w968) -> (w966:T1)
                n670 = Delete From Array(array=w973, index=w971) -> (array with subset deleted=w974:cluster{"XY Graph":cluster{dbl, dbl}[]}[])  [unwired: 1 in, 1 out]
                n671 = property on="XY Graph" class="XYGraph (strict)"("Value"=w974) -> ()  [unwired: 2 in, 2 out]
                n672 = local write "Polar Property"(w966) -> ()
              }
            }
            n673 = property on="XY Graph" class="XYGraph (strict)"("CrsrList"=T5 [] ("Cursor List")) -> ()  [unwired: 2 in, 2 out]
          }
          frame "ShowAll" {
            # "From frequency popup menu, Remove all frequency."
            n674 = Unbundle By Name(w976) -> ("Discrete/Rannge"=w975:u16)
            n675 = case shown="0, Default" w975 {
              frame 0, Default {
                n676 = property on="XY Graph" class="XYGraph (strict)"() -> ("CrsrList"=w977:T5)  [unwired: 2 in, 2 out]
                n677 = for {
                  tunnel: w977 -> [_] mode=indexing
                  i -> [w979]
                  n678 = property on="XY Graph" class="XYGraph (strict)"("Active Cursor"=w979, "Cursor.Visible"=TRUE) -> ()  [unwired: 2 in, 2 out]
                }
              }
              frame 1 {
              }
            }
          }
          frame "Invert" {
            n679 = Unbundle By Name(w981) -> ("Discrete/Rannge"=w980:u16)
            n680 = case shown="0, Default" w980 {
              frame 0, Default {
                n681 = property on="XY Graph" class="XYGraph (strict)"() -> ("CrsrList"=w982:T5)  [unwired: 2 in, 2 out]
                n682 = for {
                  tunnel: w982 -> [_] mode=indexing
                  i -> [w985]
                  n683 = property on="XY Graph" class="XYGraph (strict)"("Active Cursor"=w985) -> ("Cursor.Visible"=w984:bool)  [unwired: 2 in, 2 out]
                  n684 = Not(x=w984) -> (.not. x?=w983:bool)
                  n685 = property on="XY Graph" class="XYGraph (strict)"("Active Cursor"=w985, "Cursor.Visible"=w983) -> ()  [unwired: 2 in, 2 out]
                }
              }
              frame 1 {
              }
            }
          }
          frame "Range" {
            w1009 = T12 {"Name"="", "Color"=0, "Style"=2, "Point Style"=0, "Name Visible"=TRUE, "Allow Drag"=TRUE, "Cursor Mode"=0, "Plot"=0, "Index"=0, "Position"={"X"=0.0, "Y"=0.0}, "X Scale"=0, "Y Scale"=0, "Watch Plots"=[], "Watch All Plots"=FALSE, "Plot Area"=0, "Label Offset"={"X"=0.0, "Y"=0.2}} ("new element/subarray")
            n686 = Unbundle By Name(w1023) -> ("Show Name"=w991:bool, "CurIndex"=w1017:u16, "CurColors"=w1019:u32[], "CurValues"=w1022:dbl[])
            n687 = property on="XY Graph" class="XYGraph (strict)"("ActYScl"=0 ("Active Y Scale")) -> ("YScale.Increment"=w1025:dbl, "YScale.Minimum"=w1024:dbl)  [unwired: 2 in, 2 out]
            n688 = Increment(x=w1017) -> (x+1=w1016:u16)
            n689 = Subtract(x=w1024, y=w1025) -> (x-y=w1005:dbl)
            n690 = Multiply(x=w1025, y=2.0) -> (x*y=w1004:dbl)
            n691 = Index Array(array=w1022, index #1=w1017, index #2=w1016) -> (element #1=w988:dbl, element #2=w987:dbl)
            n692 = Index Array(array=w1019, index #1=w1017, index #2=w1016) -> (element #1=w1018:u32, element #2=w1006:u32)
            n693 = Add(x=w988, y=0.5) -> (x+y=w998:dbl)
            n694 = Add(x=w987, y=0.5) -> (x+y=w996:dbl)
            n695 = Round Toward -Infinity(1:w998) -> (0:w997:dbl)
            n696 = Round Toward -Infinity(1:w996) -> (0:w994:dbl)
            n697 = Format Value(format string="%.0f" ("string"), value (0)=w994) -> (output string=w1007:string)  [unwired: 1 in]
            n698 = Format Value(format string="%.0f" ("string"), value (0)=w997) -> (output string=w1013:string)  [unwired: 1 in]
            n699 = Bundle By Name(cluster=w1009, "Name"=w1013, "Color"=w1018, "Position.X"=w988, "Position.Y"=w1005, "Label Offset.Y"=w1004) -> (w1003:T12)
            n700 = Bundle By Name(cluster=w1009, "Name"=w1007, "Color"=w1006, "Position.X"=w987, "Position.Y"=w1005, "Label Offset.Y"=w1004) -> (w1002:T12)
            n701 = Less Or Equal?(x=w988, y=w987) -> (x <= y?=w986:bool)
            n702 = property on="XY Graph" class="XYGraph (strict)"("CrsrList"=T5 [] ("Cursor List")) -> (error out=w1000:errorcluster)  [unwired: 2 in, 1 out]
            n703 = Build Array(w1003, w1002) -> (w1001:T17)
            n704 = property on="XY Graph" class="XYGraph (strict)"(error in=w1000, "CrsrList"=w1001) -> (error out=w1020:errorcluster)  [unwired: 1 in, 1 out]
            n705 = property on="XY Graph" class="XYGraph (strict)"(error in=w1020, "Active Cursor"=u32 0, "Cursor.LineWidth"=u8 2 ("Cursor.Line Width"), "Active Cursor"=u32 1, "Cursor.LineWidth"=u8 2 ("Cursor.Line Width")) -> (error out=w989:errorcluster)  [unwired: 1 in, 1 out]
            n706 = Select(t="ShowName" ("Value (Signaling)"), s=w991, f="HideName" ("Value (Signaling)")) -> (s? t:f=w990:string)
            n707 = property on="XYCursor" class="Str"(error in=w989, "Val(Sgnl)"=w990) -> ()  [unwired: 1 in, 2 out]
            n708 = case shown="True" w986 {
              tunnel: w989 -> [_ w1028]
              frame False {
              }
              frame True {
                n709 = property on="XYCursor" class="Str"(error in=w1028, "Val(Sgnl)"="Fill" ("Value (Signaling)")) -> ()  [unwired: 1 in, 2 out]
              }
            }
          }
          frame "Discrete" {
            n710 = Unbundle By Name(w1042) -> ("Show Name"=w1033:bool, "CurColors"=w1040:u32[], "CurValues"=w1041:dbl[])  [unwired: 1 out]
            n711 = property on="XY Graph" class="XYGraph (strict)"("CrsrList"=T5 [] ("Cursor List")) -> (error out=w1037:errorcluster)  [unwired: 2 in, 1 out]
            n712 = property on="XY Graph" class="XYGraph (strict)"(error in=w1037, "ActYScl"=0 ("Active Y Scale")) -> ("YScale.Increment"=w1044:dbl, "YScale.Minimum"=w1043:dbl)  [unwired: 1 in, 2 out]
            n713 = Subtract(x=w1043, y=w1044) -> (x-y=w1039:dbl)
            n714 = Multiply(x=w1044, y=2.0) -> (x*y=w1038:dbl)
            n715 = for {
              tunnel: w1041 -> [w1051] mode=indexing
              tunnel: w1040 -> [w1052] mode=indexing
              tunnel: w1039 -> [w1057]
              tunnel: w1038 -> [w1056]
              tunnel: [w1050] -> w1030 mode=indexing
              n716 = Add(x=w1051, y=0.5) -> (x+y=w1054:dbl)
              n717 = Round Toward -Infinity(1:w1054) -> (0:w1053:dbl)
              n718 = Format Value(format string="%.0f" ("string"), value (0)=w1053) -> (output string=w1059:string)  [unwired: 1 in]
              n719 = Bundle By Name(cluster=T12 {"Name"="", "Color"=0, "Style"=2, "Point Style"=0, "Name Visible"=TRUE, "Allow Drag"=TRUE, "Cursor Mode"=0, "Plot"=0, "Index"=0, "Position"={"X"=0.0, "Y"=0.0}, "X Scale"=0, "Y Scale"=0, "Watch Plots"=[], "Watch All Plots"=FALSE, "Plot Area"=0, "Label Offset"={"X"=0.0, "Y"=0.2}} ("new element/subarray"), "Name"=w1059, "Color"=w1052, "Position.X"=w1051, "Position.Y"=w1057, "Label Offset.Y"=w1056) -> (w1050:T12)
            }
            n720 = property on="XY Graph" class="XYGraph (strict)"("CrsrList"=w1030) -> ()  [unwired: 2 in, 2 out]
            n721 = for {
              tunnel: [w1047] -> w1032
              tunnel: w1030 -> [_] mode=indexing
              i -> [w1048]
              n722 = property on="XY Graph" class="XYGraph (strict)"("Active Cursor"=w1048, "Cursor.LineWidth"=u8 2 ("Cursor.Line Width")) -> (error out=w1047:errorcluster)  [unwired: 2 in, 1 out]
            }
            n723 = Select(t="ShowName" ("Value (Signaling)"), s=w1033, f="HideName" ("Value (Signaling)")) -> (s? t:f=w1034:string)
            n724 = property on="XYCursor" class="Str"(error in=w1032, "Val(Sgnl)"=w1034) -> ()  [unwired: 1 in, 2 out]
          }
          frame "DiscreteFromRange" {
            n725 = flat-sequence {
              frame #0 {
                n726 = property on="XY Graph" class="XYGraph (strict)"() -> ("Value"=w1063:cluster{"XY Graph":cluster{dbl, dbl}[]}[])  [unwired: 2 in, 2 out]
                n727 = Array Size(array=w1063) -> (size(s)=w1062:i32)
                n728 = Decrement(x=w1062) -> (x-1=w1061:i32)
                n729 = Delete From Array(array=w1063, index=w1061) -> (array with subset deleted=w1064:cluster{"XY Graph":cluster{dbl, dbl}[]}[])  [unwired: 1 in, 1 out]
                n730 = property on="XY Graph" class="XYGraph (strict)"("Value"=w1064) -> ()  [unwired: 2 in, 2 out]
              }
              frame #1 {
                n731 = property on="XYCursor" class="Str"("Val(Sgnl)"="Discrete" ("Value (Signaling)")) -> ()  [unwired: 2 in, 2 out]
              }
            }
          }
          frame "Fill" {
            n732 = Unbundle By Name(w1077) -> ("CurIndex"=w1074:u16, "CurColors"=w1075:u32[], "CurValues"=w1076:dbl[])
            n733 = property on="XY Graph" class="XYGraph (strict)"("ActYScl"=0 ("Active Y Scale")) -> ("YScale.Maximum"=w1071:dbl, "YScale.Increment"=w1066:dbl)  [unwired: 2 in, 2 out]
            n734 = Increment(x=w1074) -> (x+1=w1073:u16)
            n735 = Index Array(array=w1076, index #1=w1074, index #2=w1073) -> (element #1=w1068:dbl, element #2=w1067:dbl)
            n736 = Index Array(array=w1075, index #1=w1074, index #2=w1073) -> ()  [unwired: 2 out]
            n737 = Add(x=w1071, y=w1066) -> (x+y=w1070:dbl)
            n738 = Less Or Equal?(x=w1068, y=w1067) -> (x <= y?=w1069:bool)
            n739 = case shown="True" w1069 {
              tunnel: w1070 -> [_ w1085]
              tunnel: w1068 -> [_ w1082]
              tunnel: w1067 -> [_ w1081]
              frame False {
              }
              frame True {
                w1084 = u32 13369344
                n740 = Bundle("CurValue0 2"=w1082, w1085) -> (w1091:cluster{"CurValue0 2":dbl, dbl})  [unwired: 1 out]
                n741 = Bundle("CurValue0 2"=w1081, w1085) -> (w1090:cluster{"CurValue0 2":dbl, dbl})  [unwired: 1 out]
                n742 = Build Array(w1091, w1090) -> (w1087:cluster{"CurValue0 2":dbl, dbl}[])
                n743 = property on="XY Graph" class="XYGraph (strict)"() -> ("Value"=w1083:cluster{"XY Graph":cluster{dbl, dbl}[]}[])  [unwired: 2 in, 2 out]
                n744 = Bundle(w1087) -> (w1086:cluster{cluster{"CurValue0 2":dbl, dbl}[]})  [unwired: 1 in]
                n745 = Array Size(array=w1083) -> (size(s)=w1080:i32)
                n746 = Insert Into Array(array=w1083, new element=w1086) -> (w1088:cluster{"XY Graph":cluster{dbl, dbl}[]}[])  [unwired: 1 in]
                n747 = property on="XY Graph" class="XYGraph (strict)"("Value"=w1088) -> (error out=w1078:errorcluster)  [unwired: 2 in, 1 out]
                n748 = for {
                  N: w1080 -> [_]
                  tunnel: [w1094] -> w1079
                  tunnel: w1078 -> [w1092]
                  i -> [w1093]
                  n749 = property on="XY Graph" class="XYGraph (strict)"(error in=w1092, "Active Plot"=w1093, "Plot.Fill To"=i16 -1) -> (error out=w1094:errorcluster)  [unwired: 1 in, 1 out]
                }
                n750 = property on="XY Graph" class="XYGraph (strict)"(error in=w1079, "Active Plot"=w1080, "Plot.Fill To"=i16 -3, "Plot.Fill/Pt. Color"=w1084, "Plot.Plot Color"=w1084) -> ()  [unwired: 1 in, 2 out]
              }
            }
          }
          frame "ShowName" {
            n751 = property on="XY Graph" class="XYGraph (strict)"() -> ("CrsrList"=w1097:T5)  [unwired: 2 in, 2 out]
            n752 = for {
              tunnel: w1097 -> [w1100] mode=indexing
              tunnel: [w1098] -> w1096 mode=indexing
              n753 = Bundle By Name(cluster=w1100, "Name Visible"=TRUE) -> (w1098:T12)
            }
            n754 = property on="XY Graph" class="XYGraph (strict)"("CrsrList"=w1096) -> ()  [unwired: 2 in, 2 out]
          }
          frame "HideName" {
            n755 = property on="XY Graph" class="XYGraph (strict)"() -> ("CrsrList"=w1102:T5)  [unwired: 2 in, 2 out]
            n756 = for {
              tunnel: w1102 -> [w1105] mode=indexing
              tunnel: [w1103] -> w1101 mode=indexing
              n757 = Bundle By Name(cluster=w1105, "Name Visible"=FALSE) -> (w1103:T12)
            }
            n758 = property on="XY Graph" class="XYGraph (strict)"("CrsrList"=w1101) -> ()  [unwired: 2 in, 2 out]
          }
          frame "NamePlot" {
            n759 = property on="XY Graph" class="XYGraph (strict)"("ActYScl"=0 ("Active Y Scale")) -> ("YScale.Increment"=w1111:dbl, "YScale.Minimum"=w1110:dbl)  [unwired: 2 in, 2 out]
            n760 = Subtract(x=w1110, y=w1111) -> (x-y=w1108:dbl)
            n761 = Multiply(x=w1111, y=2.0) -> (x*y=w1109:dbl)
            n762 = property on="XY Graph" class="XYGraph (strict)"() -> ("CrsrList"=w1107:T5)  [unwired: 2 in, 2 out]
            n763 = for {
              tunnel: [w1117] -> w1106 mode=indexing
              tunnel: w1109 -> [w1116]
              tunnel: w1108 -> [w1115]
              tunnel: w1107 -> [w1114] mode=indexing
              n764 = Bundle By Name(cluster=w1114, "Position.Y"=w1115, "Label Offset.Y"=w1116) -> (w1117:T12)
            }
            n765 = property on="XY Graph" class="XYGraph (strict)"("CrsrList"=w1106) -> ()  [unwired: 2 in, 2 out]
          }
        }
      }
      event "XY Graph": Cursor Release {
        n766 = local read "Polar Property"() -> (w1123:T1)
        n767 = event-data() -> ("CursIdx"=w1122:i32, "CursRef"=w1124:refnum<vi>)  [unwired: 1 out]
        n768 = flat-sequence {
          tunnel: w1124 -> [w1131]
          tunnel: w1123 -> [w1129]
          tunnel: w1122 -> [w1127]
          tunnel: [w1125] -> w1121
          tunnel: [w1127] -> w1119
          tunnel: [w1126] -> w1118
          tunnel: w1121 -> [w1195]
          tunnel: w1119 -> [w1192]
          tunnel: w1118 -> [w1190]
          frame #0 {
            n769 = Unbundle By Name(w1129) -> ("Discrete/Rannge"=w1125:u16, "CurValues"=w1130:dbl[], "CurIndex"=w1128:u16)
            n770 = case shown="1" w1125 {
              tunnel: w1131 -> [w1144 w1148]
              tunnel: w1130 -> [w1143 w1150]
              tunnel: w1129 -> [w1142 w1152]
              tunnel: w1128 -> [_ w1146]
              tunnel: w1127 -> [w1132 w1145]
              tunnel: [w1133 w1151] -> w1126
              frame 0, Default {
                n771 = property class="Curs"(reference=w1144) -> (reference out=w1135:refnum<vi>, "Cursor X"=w1140:dbl)  [unwired: 1 in, 1 out]
                n772 = Add(x=w1140, y=0.5) -> (x+y=w1138:dbl)
                n773 = Replace Array Subset(array=w1143, new element=w1140, index=w1132) -> (w1141:dbl[])
                n774 = Round Toward -Infinity(1:w1138) -> (0:w1137:dbl)
                n775 = Bundle By Name(cluster=w1142, "CurValues"=w1141) -> (w1134:T1)
                n776 = Format Value(format string="%.0f" ("string"), value (0)=w1137) -> (output string=w1133:string)  [unwired: 1 in]
                n777 = local write "Polar Property"(w1134) -> ()
                n778 = property class="Curs"(reference=w1135, "Cursor Name"=w1133) -> ()  [unwired: 1 in, 2 out]
              }
              frame 1 {
                n779 = Add(x=w1145, y=w1146) -> (x+y=w1147:i32)
                n780 = case shown="1" w1145 {
                  tunnel: w1150 -> [w1159 w1166]
                  tunnel: [w1157 w1164] -> w1149
                  tunnel: w1147 -> [w1156 w1161]
                  tunnel: w1148 -> [w1155 w1163]
                  frame 0, Default {
                    n781 = property class="Curs"(reference=w1155) -> ("Cursor X"=w1153:dbl)  [unwired: 1 in, 2 out]
                    n782 = Increment(x=w1156) -> (x+1=w1154:i32)
                    n783 = Index Array(array=w1159, index=w1154) -> (element=w1158:dbl)
                    n784 = Greater Or Equal?(x=w1158, y=w1153) -> (x >= y?=w1157:bool)
                  }
                  frame 1 {
                    n785 = Decrement(x=w1161) -> (x-1=w1160:i32)
                    n786 = property class="Curs"(reference=w1163) -> ("Cursor X"=w1162:dbl)  [unwired: 1 in, 2 out]
                    n787 = Index Array(array=w1166, index=w1160) -> (element=w1165:dbl)
                    n788 = Less Or Equal?(x=w1165, y=w1162) -> (x <= y?=w1164:bool)
                  }
                }
                n789 = case shown="True" w1149 {
                  tunnel: w1148 -> [w1179 w1182]
                  tunnel: w1152 -> [w1178 _]
                  tunnel: w1147 -> [w1169 w1183]
                  tunnel: [w1168 w1185] -> w1151
                  tunnel: w1150 -> [w1167 w1184]
                  frame True {
                    n790 = property class="Curs"(reference=w1179) -> (reference out=w1171:refnum<vi>, "Cursor X"=w1176:dbl)  [unwired: 1 in, 1 out]
                    n791 = Add(x=w1176, y=0.5) -> (x+y=w1174:dbl)
                    n792 = Replace Array Subset(array=w1167, new element=w1176, index=w1169) -> (w1177:dbl[])
                    n793 = Round Toward -Infinity(1:w1174) -> (0:w1173:dbl)
                    n794 = Bundle By Name(cluster=w1178, "CurValues"=w1177) -> (w1170:T1)
                    n795 = Format Value(format string="%.0f" ("string"), value (0)=w1173) -> (output string=w1168:string)  [unwired: 1 in]
                    n796 = local write "Polar Property"(w1170) -> ()
                    n797 = property class="Curs"(reference=w1171, "Cursor Name"=w1168) -> ()  [unwired: 1 in, 2 out]
                  }
                  frame False {
                    n798 = Index Array(array=w1184, index=w1183) -> (element=w1181:dbl)
                    n799 = property class="Curs"(reference=w1182, "Cursor X"=w1181) -> (reference out=w1180:refnum<vi>)  [unwired: 1 in, 1 out]
                    n800 = Add(x=w1181, y=0.5) -> (x+y=w1188:dbl)
                    n801 = Round Toward -Infinity(1:w1188) -> (0:w1187:dbl)
                    n802 = Format Value(format string="%.0f" ("string"), value (0)=w1187) -> (output string=w1185:string)  [unwired: 1 in]
                    n803 = property class="Curs"(reference=w1180, "Cursor Name"=w1185) -> ()  [unwired: 1 in, 2 out]
                  }
                }
              }
            }
          }
          frame #1 {
            n804 = flat-sequence {
              tunnel: w1195 -> [w1197]
              tunnel: [w1197] -> w1193
              tunnel: [w1196] -> w1191
              tunnel: w1190 -> [w1196]
              tunnel: [w1202] -> w1194
              tunnel: w1193 -> [w1202]
              tunnel: w1192 -> [w1204]
              tunnel: w1191 -> [w1203]
              tunnel: w1194 -> [w1216]
              frame #0 {
                n805 = case shown="1" w1197 {
                  frame 0, Default {
                  }
                  frame 1 {
                    n806 = local write "PropertyLoading"(TRUE ("PropertyLoading")) -> ()
                  }
                }
              }
              frame #1 {
                n807 = control-ref of="This VI"() -> (w1199:refnum<vi>)
                n808 = call "CRYPlot Polar Graph.vi"("pGraph VI In"=w1199, "sOption"="Replot") -> ("Freq Color"=w1200:u32[], "Freq Name"=w1201:string[])  [unwired: 6 in, 2 out]
                n809 = case shown="1" w1202 {
                  tunnel: w1204 -> [w1209 _]
                  tunnel: w1203 -> [w1208 _]
                  tunnel: w1201 -> [_ w1214]
                  tunnel: w1200 -> [_ w1213]
                  tunnel: w1199 -> [_ w1212]
                  frame 0, Default {
                    n810 = property on="Frequency" class="MCListbox (strict)"() -> ("ItemNames"=w1211:string[][])  [unwired: 2 in, 2 out]
                    n811 = Build Array(w1208, "") -> (w1206:string[])
                    n812 = Replace Array Subset(array=w1211, new element=w1206, index (row)=w1209) -> (w1210:string[][])  [unwired: 1 in]
                    n813 = property on="Frequency" class="MCListbox (strict)"("ItemNames"=w1210) -> ()  [unwired: 2 in, 2 out]
                  }
                  frame 1 {
                    n814 = call "CRYData View Legend New Insert.vi"("Color Array"=w1213, "ItemName Array"=w1214, "sOption"="POLAR_XY", "pGraph VI In"=w1212) -> ()  [unwired: 7 in, 1 out]
                  }
                }
              }
              frame #2 {
                n815 = case shown="1" w1216 {
                  frame 0, Default {
                  }
                  frame 1 {
                    n816 = local write "PropertyLoading"(FALSE ("PropertyLoading")) -> ()
                  }
                }
              }
            }
            n817 = case shown="1" w1195 {
              frame 0, Default {
              }
              frame 1 {
                n818 = property on="XY Graph" class="XYGraph (strict)"() -> ("Value"=w1221:cluster{"XY Graph":cluster{dbl, dbl}[]}[])  [unwired: 2 in, 2 out]
                n819 = Array Size(array=w1221) -> (size(s)=w1220:i32)
                n820 = Decrement(x=w1220) -> (x-1=w1219:i32)
                n821 = Delete From Array(array=w1221, index=w1219) -> (array with subset deleted=w1222:cluster{"XY Graph":cluster{dbl, dbl}[]}[])  [unwired: 1 in, 1 out]
                n822 = property on="XY Graph" class="XYGraph (strict)"("Value"=w1222) -> (error out=w1218:errorcluster)  [unwired: 2 in, 1 out]
                n823 = property on="XYCursor" class="Str"(error in=w1218, "Val(Sgnl)"="Fill" ("Value (Signaling)")) -> ()  [unwired: 1 in, 2 out]
              }
            }
          }
        }
        n824 = property on="Repaint Watermark" class="DigNum (strict)"("Val(Sgnl)"=-1 ("Value (Signaling)")) -> ()  [unwired: 2 in, 2 out]
      }
      event "XY Graph": Scale Range Change {
        n825 = event-data() -> ()  [unwired: 4 out]
        n826 = property on="XYCursor" class="Str"("Val(Sgnl)"="NamePlot" ("Value (Signaling)")) -> ()  [unwired: 2 in, 2 out]
      }
      event "Polar Plot", "XY Graph": Drag Enter {
        n827 = event-data() -> ("Available Data Names"=w1226:string[])  [unwired: 1 out]
        n828 = disable-structure shown="Disabled" {
          disable-tunnel: w1226 -> [w1228 _]
          disable-tunnel: [w1227 TRUE] -> w1225
          frame Disabled {
            n829 = Search 1D Array(1D array=w1228, element="CRY_GRAPH_DATA") -> (index of element=w1230:i32)  [unwired: 1 out]
            n830 = Not Equal?(x=w1230, y=-1) -> (x != y?=w1227:bool)
          }
          frame Enabled {
          }
        }
        n831 = event-data("Accepted?"=w1225) -> ()  [unwired: 1 in, 1 out]
      }
      event "Polar Plot", "XY Graph": Drop {
        n832 = event-data() -> ()  [unwired: 2 out]
        n833 = local read "Event Name"() -> (w1233:string)
        n834 = local read "TotalPlot"() -> (w1237:u32)
        n835 = control-ref of="This VI"() -> (w1234:refnum<vi>)
        n836 = call "CRYDrop Data in Same Graph.vi"("pGraph VI"=w1234, "Queue"=w1235, "Total Plot In"=w1237, "sAction"=w1233) -> ("Accepted?"=w1236:bool, "Total Plot Out"=w1238:u32)  [unwired: 3 in, 3 out]
        n837 = local write "TotalPlot"(w1238) -> ()
        n838 = event-data("Accepted?"=w1236) -> ()  [unwired: 1 in, 1 out]
      }
    }
    n839 = global read "CRYMain Sub Window Global.vi" "gStop"() -> (w139:bool)
    n840 = Or(x=w139, y="stop") -> (x .or. y?=w134:bool)
  }
  n841 = flat-sequence {
    tunnel: w7 -> [_]
    frame #0 {
      n842 = local write "StateOut"(TRUE ("StateOut")) -> ()
    }
  }
